vi "MC_7_12c_JW.vi"() -> ()   [LabVIEW 2011]
uses:
  <vilib>/Utility/file.llb/Read From Spreadsheet File (string).vi
  <vilib>/regexp/Match Regular Expression.xnode
  <vilib>/Utility/file.llb/Write To Spreadsheet File (string).vi
  <vilib>/Utility/file.llb/Write To Spreadsheet File (DBL).vi
  <vilib>/Utility/inputDevices.llb/keyboardAcquire.vi
panel:
  out "Rec: Temp":dbl
  out "Date Created":string
  out "Comments":string
  out "Folder Index":dbl caption="Length"
  out "Current \nRecord":string[](array[string])
  out "Transformer \nHeaders":string[](array[string])
  out "Current Device ID":string
  out "Column":string
  out "Row":string
  out "Rec: Concentration":dbl
  out "Rec: Solvent":string
  out "Rec: Method":string
  in  "?":T1(tab)
  out "Rec: Material":string
  in  "Treatment Concentration (mM):":dbl=30.0
  in  "Surface Treatment:":string
  in  "# Drops*:":dbl=inf
  in  "Solution Temp (C):":dbl=55.0
  in  "Relative Humidity (%):":dbl=nan
  in  "Room Temp (F):":dbl=nan
  in  "Time (s):":dbl=80.0
  out "Accel (RPM/s):":dbl
  in  "RPM:":dbl=1000.0
  in  "Wait Time (s):":dbl=10.0
  in  "Sample #:":dbl=1.0
  in  "Fabricator:":string="Jeremy"
  in  "Data File":path
  out "Data Folder":path
  in  "Image Folder":path
  out "Image File":path=path "D:/UserData/Desktop/Jeremy/WFU/Research/Programs/VI mods/Image Not Found.png"
  in  "Ramp (s):":dbl=3.0
  out "Calc: Trap Density-STS":dbl format="%#_4e"
  out "New: Trap Density-STS":dbl format="%#_4e"
  out "Rec: Trap Density-STS":dbl caption="Trap Density-STS" format="%#_4e"
  out "Calc: Trap Density-VT":dbl format="%#_4e"
  out "New: Trap Density-VT":dbl format="%#_4e"
  out "Rec: Trap Density-VT":dbl caption="Trap Density-VT" format="%#_4e"
  out "Calc: Onset V":dbl
  out "New: Onset":dbl
  out "Rec: Onset V":dbl caption="Onset V"
  out "Calc: Mobility-Lin":dbl format="%#_4e"
  out "New: Mobility-Lin":dbl format="%#_4e"
  out "Rec: Mobility-Lin":dbl caption="Mobility-Lin" format="%#_4e"
  out "Calc: Mobility-Sat":dbl format="%#_4e"
  out "Rec: Length":dbl caption="Length"
  out "Rec: Width":dbl caption="Width"
  out "Rec: Dielectric (d)":dbl caption="Dielectric (d)"
  out "XY Graph":cluster{dbl[], dbl[]}[](graph)
  in  "NumPts":dbl=5.0
  in  "Cancel Button":bool
  in  "Next Button":bool
  in  "Previous Button":bool
  in  "Up Button":bool
  in  "Down Button":bool
  out "Data Name":string
  in  "Save Changes?":bool
  in  "New: Dielectric":dbl
  in  "New: Length":dbl
  in  "New: Width":dbl
  out "New: Mobility-Sat":dbl format="%#_4e"
  in  "Slide":dbl(slide) step=1.0 scale=-14.3..84.0 scale format="%#_1p"
  in  "Blank Button":bool
  in  "Zoom":i16(slide)=-3 scale=-5.0..5.0
  out "Image Out 2":T2(plugin-control)
  out "Image Out":T2(plugin-control)
  in  "Magnification":u16(ring) items=["5x", "10x", "20x", "50x", "80x"]
  out "Total Width":dbl
  out "Distances":dbl[](array[numeric])
  in  "Undo Button":bool
  in  "Remove Button":bool
  out "Rec: Mobility-Sat":dbl caption="Mobility-Sat" format="%#_4e"
  out "Index":string
  out "Image Name":string
  in  "Export":bool
  out "Calc: VT":dbl
  out "New: VT":dbl
  in  "Manual":bool
  out "XY Graph 2":cluster{dbl[], dbl[]}[](graph)
  in  "Next Button 2":bool
  in  "Previous Button 2":bool
  in  "Slide 2":dbl(slide) step=1.0 scale=-1.0..82.0 scale format="%#_1p"
  out "Calc: STS":dbl
  out "New: STS":dbl
  in  "NumPts 2":dbl=5.0 caption="NumPts"
  out "Rec: VT":dbl caption="Threshold V"
  out "Rec: STS":dbl caption="STS"
  out "Rec: On/Off":dbl caption="On/Off" format="%#_3e"
  in  "Save Changes? 2":bool
  in  "Save Changes? 3":bool
  out "Date Recorded":string="Date Recorded"
  out "String":string
  in  "No Image":path=path "D:/UserData/Desktop/Jeremy/WFU/Research/Programs/VI mods/Image Not Found.png"
  in  "Project":path=path "D:/UserData/Desktop/Jeremy/WFU/Research/Programs/Mega Awesome/DeviceData.opj"
  out "Index 2":dbl
  out "Array 8":dbl[](array[numeric])
  out "Array 7":dbl[](array[numeric])
  out "ROI Descriptor out":T3 {"Contours"."Type" items=["No Selection", "Point", "Line", "Rectangle", "Oval", "Polygon", "Freehand Region", "Annulus", "Unused2", "Unused3", "Broken Line", "Freehand Line", "Rotated Rectangle"]}
  out "ROI Descriptor":T3 {"Contours"."Type" items=["No Selection", "Point", "Line", "Rectangle", "Oval", "Polygon", "Freehand Region", "Annulus", "Unused2", "Unused3", "Broken Line", "Freehand Line", "Rotated Rectangle"]}
  out "Numeric 3":dbl
  out "Array 6":dbl[][](array[numeric])
  out "Cluster":T4
  out "Array 5":dbl[](array[numeric])
  out "Array 4":dbl[](array[numeric])
  out "Array 3":dbl[](array[numeric])
  out "Numeric 2":dbl
  out "Numeric":dbl
  out "Array 2":dbl[](array[numeric])
  out "Array":dbl[](array[numeric])
  out "Device Index":dbl
  out "Table Control 2":string[][](table)
  out "Table Control":string[][](table)
  in  "Row Start":dbl=20.0
  # "Data Locations"
  # "Data Location"
  # "Image Location"
  # "Sample Properties"
  # "*     Inf = Full coverage\n   NaN = Unknown or Not Applicable"
  # "Recorded"
  # "Calculated"
  # "Re-Calculated"
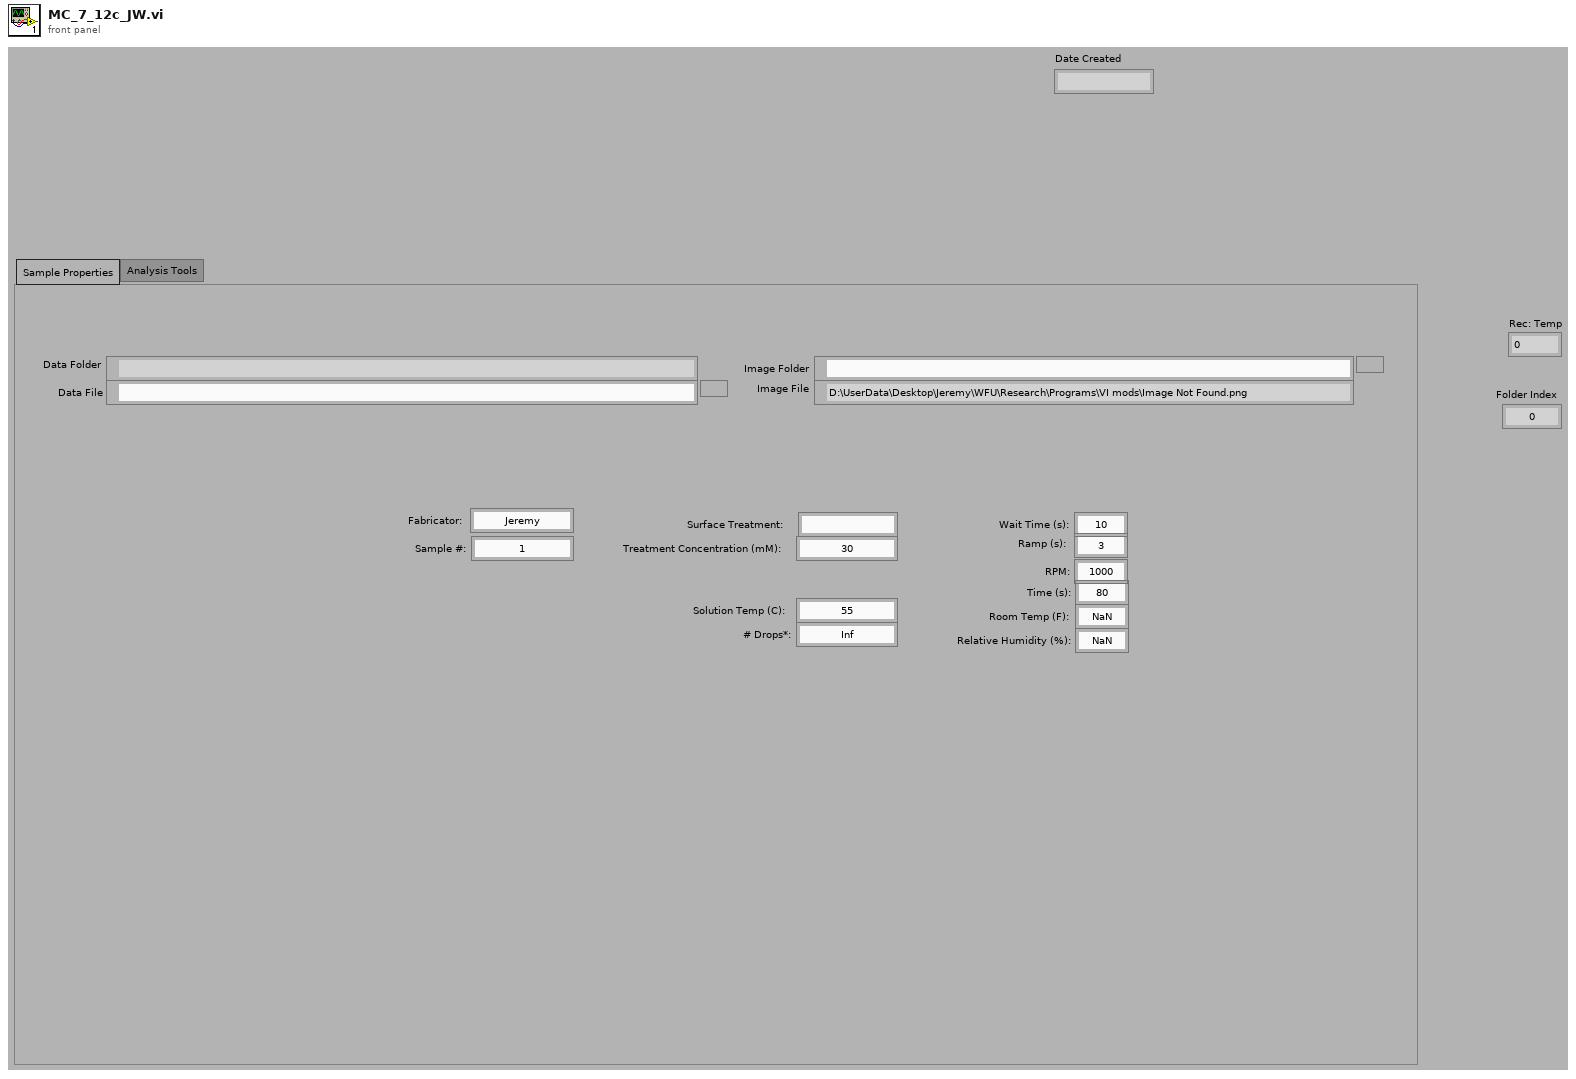
[diagram p1: front panel]
types:
  T1 = enum32{"Sample Properties", "Analysis Tools", "Current Database"}
  T2 = typedef "IMAQ Image.ctl" = refnum<image>
  T3 = typedef "ROI Descriptor" = cluster{"Global Rectangle":i32[], "Contours":cluster{"ID":enum32{"External", "Internal"}, "Type":u32, "Coordinates":i32[]}[]}
  T4 = cluster{"Numeric":dbl, "Numeric 2":dbl, "Numeric 3":dbl, "Numeric 4":dbl}
  T5 = cluster{"Mobility-Sat":dbl, "Moblitity-Lin":dbl, "On/Off":dbl, "Threshold Voltage":dbl, "Onset Voltage":dbl, "STS":dbl, "Trap Density-VT":dbl, "Trap Density-STS":dbl}
  T6 = cluster{"Date Recorded":string, "Index":string, "Length":dbl, "Width":dbl, "Sample Temp":dbl}
  T7 = cluster{"Date Created":string, "Material":string, "Solvent":string, "Concentration":dbl, "Method":string, "Dielectric (nm)":dbl, "Treatment":string, "Comments":string}
  T8 = cluster{"[0]":cluster{dbl[], dbl[]}, "[1]":cluster{dbl[], dbl[]}, "[2]":cluster{dbl[], dbl[]}, "[3]":cluster{dbl[], dbl[]}, "[4]":cluster{dbl[], dbl[]}, "[5]":cluster{dbl[], dbl[]}, "[6]":cluster{dbl[], dbl[]}, "[7]":cluster{dbl[], dbl[]}, "[8]":cluster{dbl[], dbl[]}}
  T9 = cluster{"Global Rectangle":i32[], "Contours":cluster{"Contour Type":u32, "ROI Type":u32, "Points":i32[]}[]}
  T10 = typedef "LVBoundsTypeDef.ctl" = cluster{"Width":u32, "Height":u32}
  T11 = enum16{"0", "1", "2", "3", "4", "5", "6", "7", "8", "9", "A", "B", "C", "D", "E", "F", "G", "H", "I", "J", "K", "L", "M", "N", "O", "P", "Q", "R", "S", "T", "U", "V", "W", "X", "Y", "Z", "F1", "F2", "F3", "F4", "F5", "F6", "F7", "F8", "F9", "F10", "F11", "F12", "F13", "F14", "F15", "ADD", "BACK", "BACKSLASH", "CAPITAL", "COMMA", "DECIMAL", "DELETE", "DIVIDE", "DOWN", "END", "EQUALS", "ESCAPE", "GRAVE (`)", "HOME", "INSERT", "LBRACKET", "LCONTROL", "LEFT", "L ALT", "LSHIFT", "LWIN", "MINUS", "MULTIPLY", "NEXT", "NUMLOCK", "NUMPAD_0", "NUMPAD_1", "NUMPAD_2", "NUMPAD_3", "NUMPAD_4", "NUMPAD_5", "NUMPAD_6", "NUMPAD_7", "NUMPAD_8", "NUMPAD_9", "PAUSE", "PERIOD", "PRIOR (PG UP)", "RBRACKET", "RCONTROL", "RETURN", "RIGHT", "R ALT", "RSHIFT", "RWIN", "SCROLL", "SEMICOLON", "SLASH", "SPACE", "SUBTRACT", "TAB", "UP", "ENTER (num pad)", "' (quote)"}[]
  T12 = cluster{"Contour Type":u32, "ROI Type":u32, "Points":i32[]}[]
  T13 = cluster{i32[], cluster{"Contour Type":u32, "ROI Type":u32, "Points":i32[]}[]}
  T14 = enum16{"0", "1", "2", "3", "4", "5", "6", "7", "8", "9", "A", "B", "C", "D", "E", "F", "G", "H", "I", "J", "K", "L", "M", "N", "O", "P", "Q", "R", "S", "T", "U", "V", "W", "X", "Y", "Z", "F1", "F2", "F3", "F4", "F5", "F6", "F7", "F8", "F9", "F10", "F11", "F12", "F13", "F14", "F15", "ADD", "BACK", "BACKSLASH", "CAPITAL", "COMMA", "DECIMAL", "DELETE", "DIVIDE", "DOWN", "END", "EQUALS", "ESCAPE", "GRAVE (`)", "HOME", "INSERT", "LBRACKET", "LCONTROL", "LEFT", "L ALT", "LSHIFT", "LWIN", "MINUS", "MULTIPLY", "NEXT", "NUMLOCK", "NUMPAD_0", "NUMPAD_1", "NUMPAD_2", "NUMPAD_3", "NUMPAD_4", "NUMPAD_5", "NUMPAD_6", "NUMPAD_7", "NUMPAD_8", "NUMPAD_9", "PAUSE", "PERIOD", "PRIOR (PG UP)", "RBRACKET", "RCONTROL", "RETURN", "RIGHT", "R ALT", "RSHIFT", "RWIN", "SCROLL", "SEMICOLON", "SLASH", "SPACE", "SUBTRACT", "TAB", "UP", "ENTER (num pad)", "' (quote)"}
  T15 = cluster{string, sgl, bool, bool, bool, bool, bool, bool, i32}
  T16 = cluster{i32, cluster{string, sgl, bool, bool, bool, bool, bool, bool, i32}, i32, i32}
  T17 = cluster{"Contour Type":u32, "ROI Type":u32, "Points":i32[]}
  T18 = cluster{"Points[0]":i32, "Points[1]":i32, "Points[2]":i32, "Points[3]":i32, "Points[4]":i32, "Points[5]":i32, "Points[6]":i32, "Points[7]":i32, "Points[8]":i32}
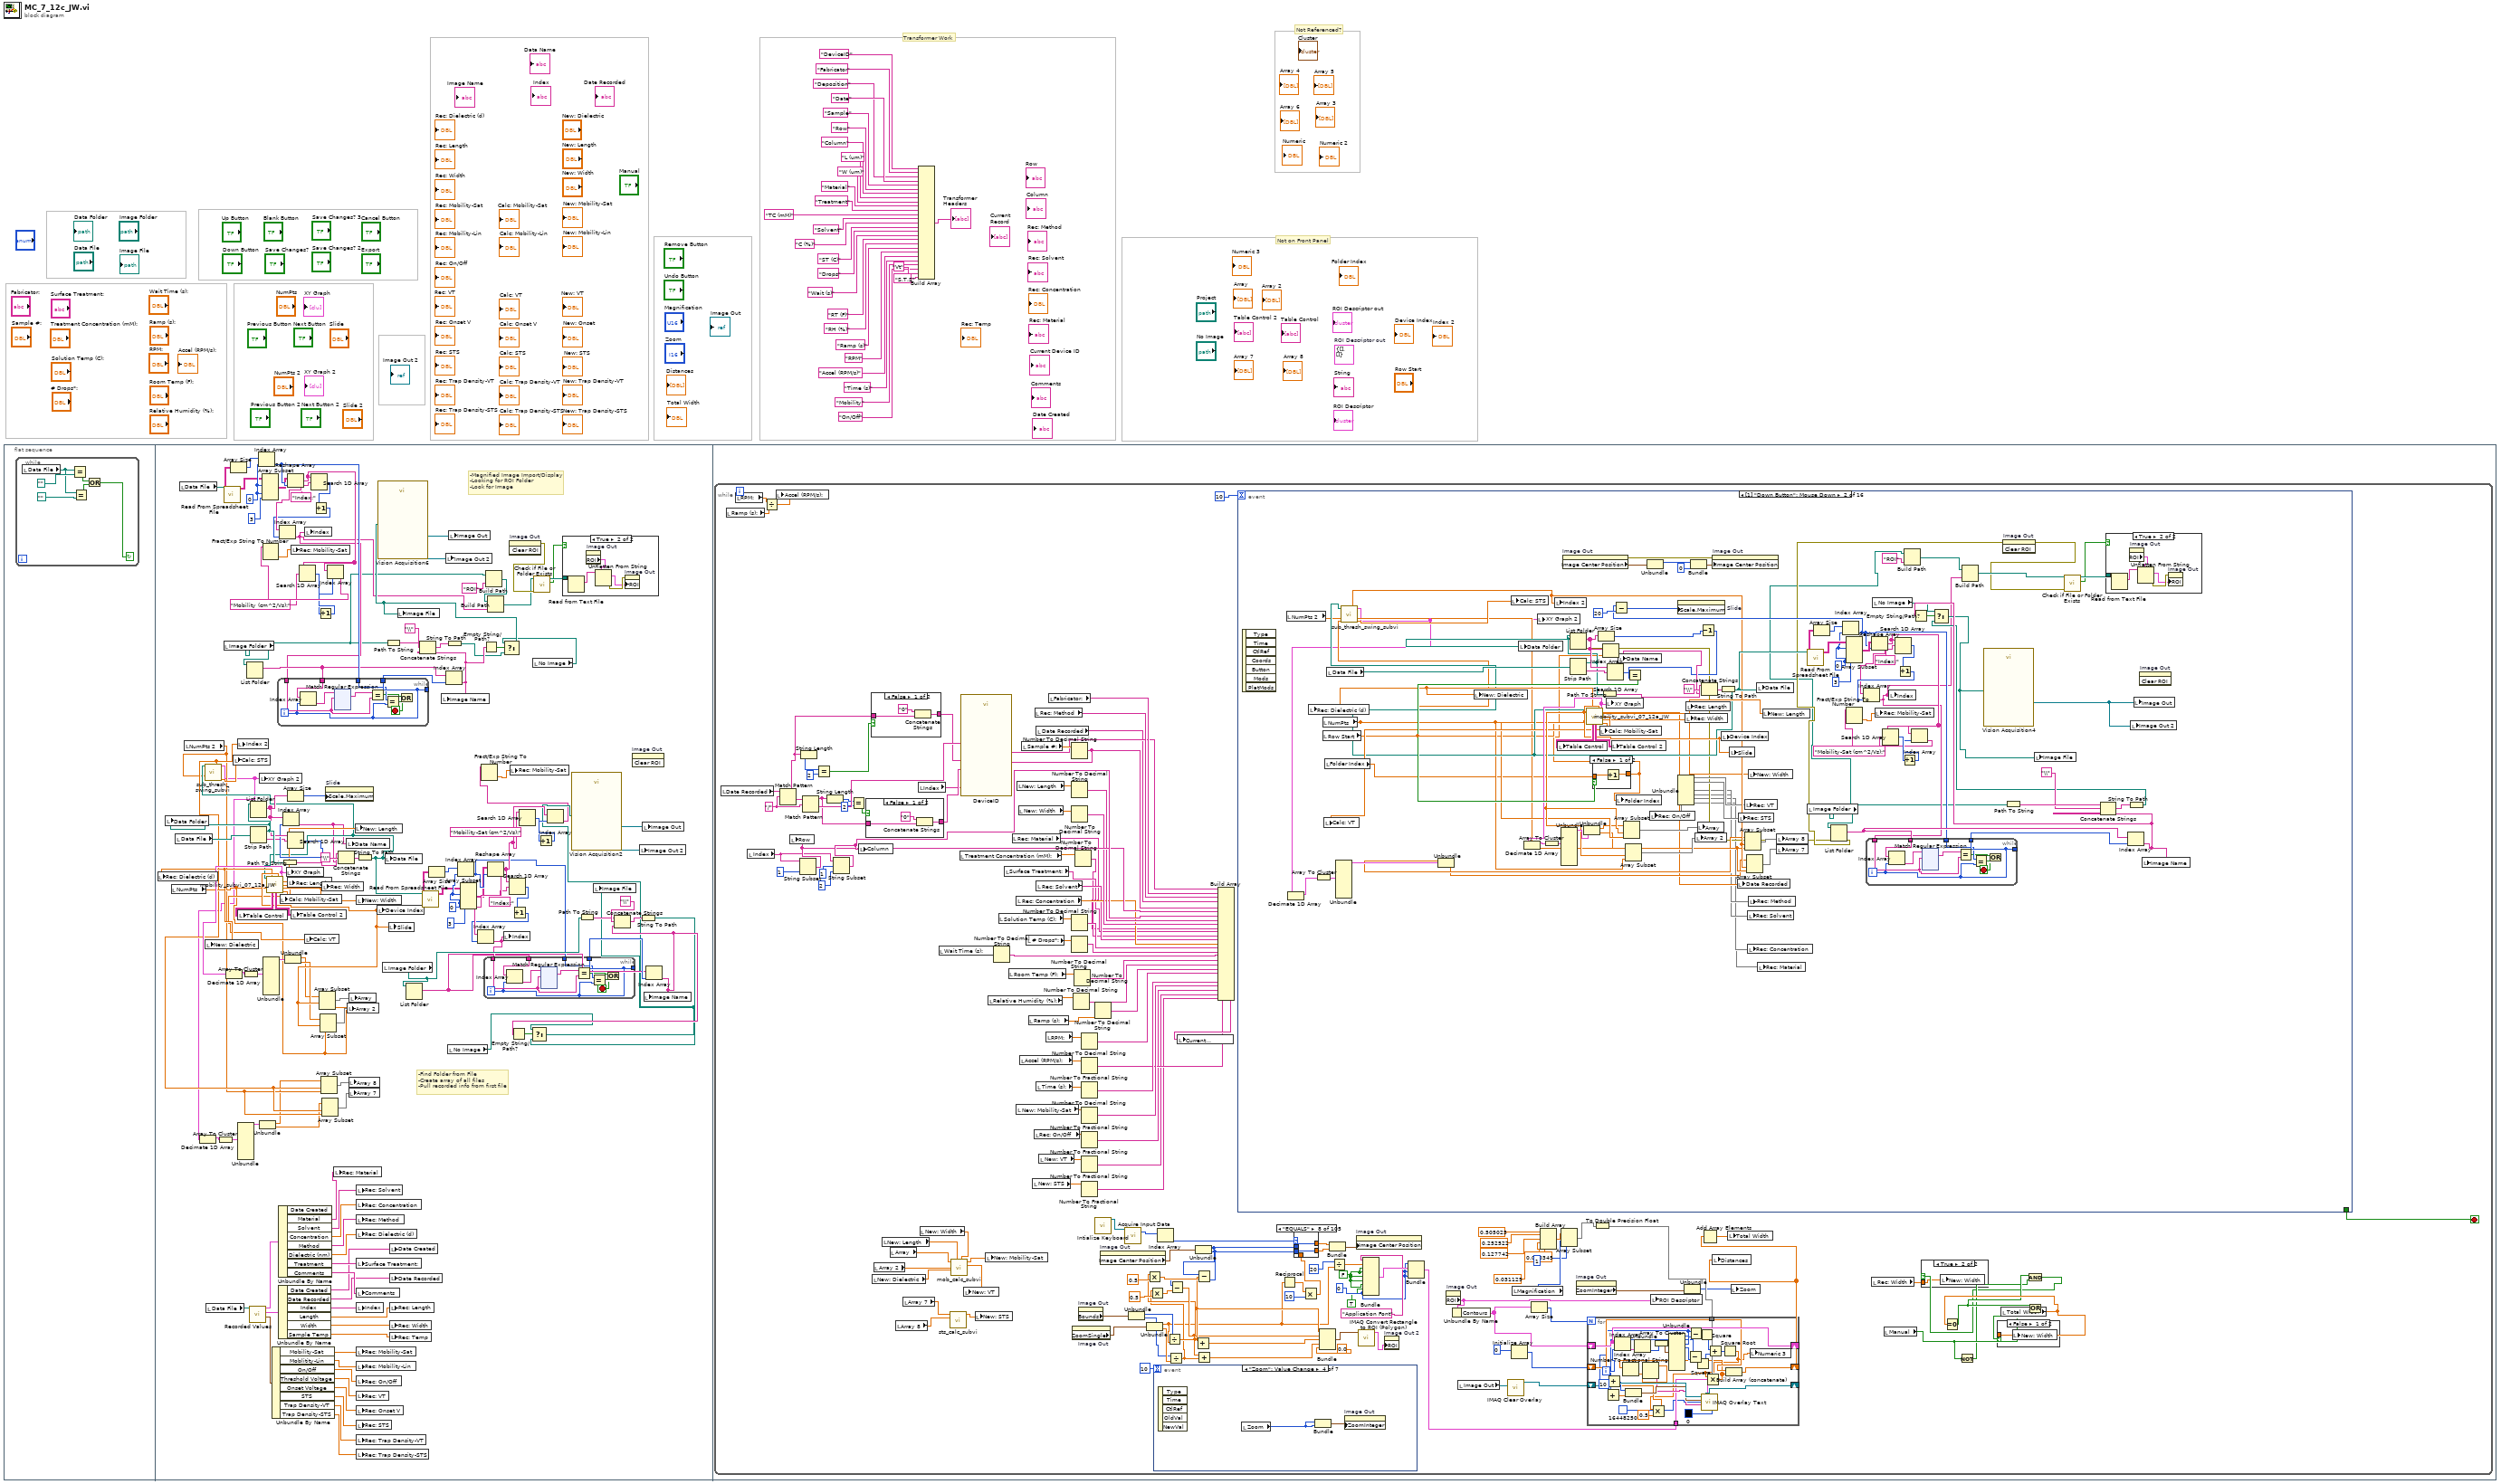
[diagram p0: block diagram]
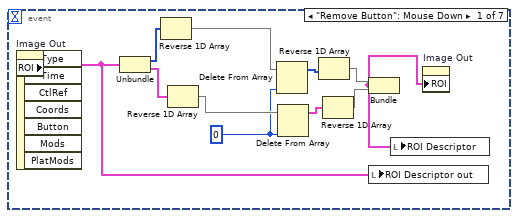
[diagram p7: hidden frame]
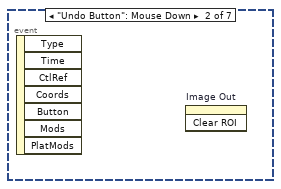
[diagram p8: hidden frame]
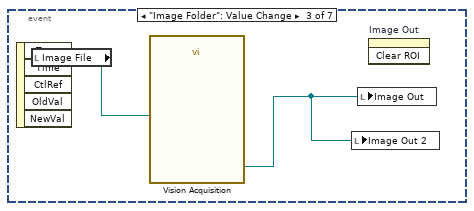
[diagram p9: hidden frame]
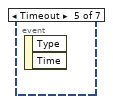
[diagram p10: hidden frame]
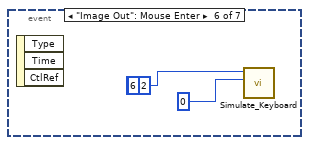
[diagram p11: hidden frame]
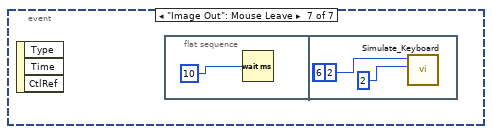
[diagram p12: hidden frame]
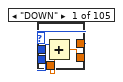
[diagram p13: hidden frame]
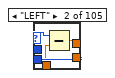
[diagram p14: hidden frame]
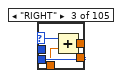
[diagram p15: hidden frame]
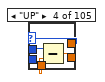
[diagram p16: hidden frame]
diagram:
  (unwired) T3 {"Global Rectangle"=[], "Contours"=[]}  # ROI Descriptor out
  # "Not Referenced?"
  # "Transformer Work"
  # "Not on Front Panel"
  n1 = flat-sequence {
    frame #0 {
      n2 = while {
        stop <- w29 continue-if-true
        n3 = local read "Data File"() -> (w31:path)
        n4 = Equal?(x=w31, y=path "") -> (x = y?=w33:bool)
        n5 = Equal?(x=w31, y=path "") -> (x = y?=w32:bool)
        n6 = Or(x=w33, y=w32) -> (x .or. y?=w29:bool)
      }
    }
    frame #1 {
      w116 = 0
      w145 = 0
      # "-Find Folder from File\n-Create array of all files\n-Pull recorded info from first file"
      # "-Magnified Image Import/Display\n-Looking for ROI Folder\n-Look for Image"
      n7 = local read "NumPts"() -> (w92:dbl)
      n8 = local read "Data File"() -> (w120:path)
      n9 = local read "Data File"() -> (w140:path)
      n10 = local read "NumPts 2"() -> (w87:dbl)
      n11 = local read "Data File"() -> (w59:path)
      n12 = call-poly <vilib>:"Read From Spreadsheet File.vi"("file path (dialog if empty)"=w140) -> ("all rows"=w143:string[][])  [unwired: 6 in, 4 out]
      n13 = local read "Image Folder"() -> (w62:path)
      n14 = Array Size(array=w143) -> (size(s)=w144:i32[])
      n15 = List Folder(path=w62) -> (filenames=w149:string[])  [unwired: 3 in, 3 out]
      n16 = call "Recorded Values.vi"("Path"=w59) -> ("Recorded Char"=w57:T5, "Recorded Prop"=w56:T6, "Fabrication Prop"=w58:T7)  [unwired: 8 in]
      n17 = Strip Path(path=w120) -> (stripped path=w121:path, name=w103:string)
      n18 = local write "Data Folder"(w121) -> ()
      n19 = List Folder(path=w121) -> (filenames=w110:string[])  [unwired: 3 in, 3 out]
      n20 = Index Array(array=w144, index=w145) -> (element=w151:i32)
      n21 = Array Subset(array=w143, index (row)=w145, index (col)=w145, length (col)=3) -> (w142:string[][])  [unwired: 1 in]
      n22 = Unbundle By Name(w57) -> ("Mobility-Sat"=w42:dbl, "Moblitity-Lin"=w41:dbl, "On/Off"=w40:dbl, "Threshold Voltage"=w39:dbl, "Onset Voltage"=w38:dbl, "STS"=w37:dbl, "Trap Density-VT"=w36:dbl, "Trap Density-STS"=w35:dbl)
      n23 = Unbundle By Name(w58) -> ("Material"=w55:string, "Solvent"=w54:string, "Concentration"=w53:dbl, "Method"=w52:string, "Dielectric (nm)"=w51:dbl, "Treatment"=w50:string, "Comments"=w49:string)  [unwired: 1 out]
      n24 = Unbundle By Name(w56) -> ("Date Created"=w48:string, "Date Recorded"=w47:string, "Index"=w46:string, "Length"=w45:dbl, "Width"=w44:dbl, "Sample Temp"=w43:dbl)
      n25 = Path To String(path=w121) -> (string=w102:string)
      n26 = Reshape Array(w142, w151) -> (w161:string[])
      n27 = Array Size(array=w110) -> (size(s)=w111:i32)
      n28 = Search 1D Array(1D array=w110, element=w103) -> (index of element=w109:i32)  [unwired: 1 in]
      n29 = Index Array(array=w110, index=w109) -> (element=w61:string)
      n30 = Search 1D Array(1D array=w161, element="Mobility (cm^2/Vs):") -> (index of element=w156:i32)  [unwired: 1 in]
      n31 = Search 1D Array(1D array=w161, element="Index:") -> (index of element=w148:i32)  [unwired: 1 in]
      n32 = Increment(x=w148) -> (x+1=w147:i32)
      n33 = Index Array(array=w161, index=w147) -> (element=w63:string)
      n34 = while {
        tunnel: w149 -> [w294]
        tunnel: w63 -> [w292]
        tunnel: [w291] -> _
        tunnel: [w291] -> w150
        tunnel: w151 -> [w290]
        i -> [w291]
        stop <- w287 stop-if-true
        n35 = Index Array(array=w294, index=w291) -> (element=w295:string)
        n36 = xnode "Match Regular Expression"("input string"=w295, "regular expression"=w292) -> ("whole match"=w293:string)  [unwired: 4 in, 4 out]
        n37 = Equal?(x=w293, y=w292) -> (x = y?=w289:bool)
        n38 = Equal?(x=w290, y=w291) -> (x = y?=w288:bool)
        n39 = Or(x=w289, y=w288) -> (x .or. y?=w287:bool)
      }
      n40 = local write "Index"(w63) -> ()
      n41 = Increment(x=w156) -> (x+1=w157:i32)
      n42 = property on="Slide" class="Slide (strict)"("Scale.Maximum"=w111) -> ()  [unwired: 2 in, 2 out]
      n43 = Index Array(array=w161, index=w157) -> (element=w159:string)
      n44 = Fract/Exp String To Number(string=w159) -> (number=w160:dbl)  [unwired: 3 in, 1 out]
      n45 = local write "Rec: Mobility-Sat"(w160) -> ()
      n46 = local write "Rec: Material"(w55) -> ()
      n47 = Concatenate Strings(w102, "\\", w61) -> (w104:string)
      n48 = local write "Data Name"(w61) -> ()
      n49 = local write "Rec: Solvent"(w54) -> ()
      n50 = local write "Rec: Concentration"(w53) -> ()
      n51 = local write "Rec: Method"(w52) -> ()
      n52 = local write "Rec: Dielectric (d)"(w51) -> ()
      n53 = local write "Surface Treatment:"(w50) -> ()
      n54 = local write "Comments"(w49) -> ()
      n55 = local write "Index"(w46) -> ()
      n56 = local write "Rec: Mobility-Sat"(w42) -> ()
      n57 = local write "Rec: Mobility-Lin"(w41) -> ()
      n58 = local write "Rec: On/Off"(w40) -> ()
      n59 = local write "Rec: VT"(w39) -> ()
      n60 = local write "Rec: Onset V"(w38) -> ()
      n61 = local write "Rec: STS"(w37) -> ()
      n62 = local write "Rec: Trap Density-VT"(w36) -> ()
      n63 = local write "Rec: Trap Density-STS"(w35) -> ()
      n64 = String To Path(string=w104) -> (path=w93:path)
      n65 = call "sub_thresh_swing_subvi.vi"("Path"=w93, "NumPts"=w87) -> ("Index"=w88:dbl, "XY Graph"=w83:cluster{dbl[], dbl[]}[], "Sub Threshold Swing"=w94:dbl)  [unwired: 9 in, 2 out]
      n66 = Decimate 1D Array(w83) -> (w84:cluster{dbl[], dbl[]}[])  [unwired: 1 out]
      n67 = Array To Cluster(array=w84) -> (cluster=w86:T8)
      n68 = local write "Calc: STS"(w94) -> ()
      n69 = local write "Index 2"(w88) -> ()
      n70 = Unbundle(w86) -> ("[0]"=w85:cluster{dbl[], dbl[]})  [unwired: 8 out]
      n71 = local write "XY Graph 2"(w83) -> ()
      n72 = Unbundle(w85) -> (w81:dbl[], w80:dbl[])
      n73 = call "mobility_subvi_07_12a_JW.vi"("Path"=w93, "NumPts"=w92) -> ("Dielectric (d)"=w98:dbl, "Index"=w99:dbl, "XY Graph"=w139:cluster{dbl[], dbl[]}[], "Length"=w97:dbl, "Vt"=w95:dbl, "Width"=w96:dbl, "Table Control"=w106:string[][], "Table Control 2"=w107:string[][], "Mobility"=w108:dbl)  [unwired: 4 in, 1 out]
      n74 = local write "Rec: Dielectric (d)"(w98) -> ()
      n75 = local write "New: Dielectric"(w98) -> ()
      n76 = Decimate 1D Array(w139) -> (w138:cluster{dbl[], dbl[]}[])  [unwired: 1 out]
      n77 = local write "Table Control"(w106) -> ()
      n78 = Array To Cluster(array=w138) -> (cluster=w136:T8)
      n79 = Unbundle(w136) -> ("[0]"=w137:cluster{dbl[], dbl[]})  [unwired: 8 out]
      n80 = local write "Calc: Mobility-Sat"(w108) -> ()
      n81 = Unbundle(w137) -> (w82:dbl[], w89:dbl[])
      n82 = local write "XY Graph"(w139) -> ()
      n83 = local write "Rec: Length"(w97) -> ()
      n84 = local write "Table Control 2"(w107) -> ()
      n85 = local write "Calc: VT"(w95) -> ()
      n86 = Array Subset(array=w82, index=w99, length=w92) -> (w100:dbl[])
      n87 = Array Subset(array=w89, index=w99, length=w92) -> (w101:dbl[])
      n88 = Array Subset(array=w81, index=w88, length=w87) -> (w91:dbl[])
      n89 = local write "Rec: Width"(w96) -> ()
      n90 = Array Subset(array=w80, index=w88, length=w87) -> (w90:dbl[])
      n91 = local write "Array 2"(w101) -> ()
      n92 = local write "Array 8"(w91) -> ()
      n93 = local write "Array 7"(w90) -> ()
      n94 = local write "Array"(w100) -> ()
      n95 = local write "New: Length"(w97) -> ()
      n96 = local write "New: Width"(w96) -> ()
      n97 = local write "Device Index"(w99) -> ()
      n98 = local read "Image Folder"() -> (w127:path)
      n99 = local write "Data File"(w93) -> ()
      n100 = Path To String(path=w62) -> (string=w153:string)
      n101 = local write "Slide"(w99) -> ()
      n102 = local write "Date Created"(w48) -> ()
      n103 = local write "Date Recorded"(w47) -> ()
      n104 = local write "Rec: Length"(w45) -> ()
      n105 = local write "Rec: Width"(w44) -> ()
      n106 = local write "Rec: Temp"(w43) -> ()
      n107 = List Folder(path=w127) -> (filenames=w123:string[])  [unwired: 3 in, 3 out]
      n108 = call-poly <vilib>:"Read From Spreadsheet File.vi"("file path (dialog if empty)"=w93) -> ("all rows"=w114:string[][])  [unwired: 6 in, 4 out]
      n109 = Array Size(array=w114) -> (size(s)=w115:i32[])
      n110 = Index Array(array=w149, index=w150) -> (element=w79:string)
      n111 = Concatenate Strings(w153, "\\", w79) -> (w154:string)
      n112 = local write "Image Name"(w79) -> ()
      n113 = String To Path(string=w154) -> (path=w77:path)
      n114 = local read "No Image"() -> (w71:path)
      n115 = Index Array(array=w115, index=w116) -> (element=w126:i32)
      n116 = Array Subset(array=w114, index (row)=w116, index (col)=w116, length (col)=3) -> (w113:string[][])  [unwired: 1 in]
      n117 = Empty String/Path?(string/path=w79) -> (empty?=w78:bool)
      n118 = Build Path(base path=w62, name or relative path="ROI") -> (appended path=w65:path)
      n119 = Build Path(base path=w65, name or relative path=w63) -> (appended path=w64:path)
      n120 = Reshape Array(w113, w126) -> (w135:string[])
      n121 = invoke on="Image Out" class="ImageControl" method="Clear ROI"() -> (error out=w69:errorcluster)  [unwired: 3 in, 2 out]
      n122 = Search 1D Array(1D array=w135, element="Index:") -> (index of element=w119:i32)  [unwired: 1 in]
      n123 = Increment(x=w119) -> (x+1=w118:i32)
      n124 = Index Array(array=w135, index=w118) -> (element=w124:string)
      n125 = while {
        tunnel: w123 -> [w174]
        tunnel: w124 -> [w172]
        tunnel: [w171] -> _
        tunnel: [w171] -> w125
        tunnel: w126 -> [w170]
        i -> [w171]
        stop <- w167 stop-if-true
        n126 = Index Array(array=w174, index=w171) -> (element=w175:string)
        n127 = xnode "Match Regular Expression"("input string"=w175, "regular expression"=w172) -> ("whole match"=w173:string)  [unwired: 4 in, 4 out]
        n128 = Equal?(x=w173, y=w172) -> (x = y?=w169:bool)
        n129 = Equal?(x=w170, y=w171) -> (x = y?=w168:bool)
        n130 = Or(x=w169, y=w168) -> (x .or. y?=w167:bool)
      }
      n131 = local write "Index"(w124) -> ()
      n132 = Search 1D Array(1D array=w135, element="Mobility-Sat (cm^2/Vs):") -> (index of element=w131:i32)  [unwired: 1 in]
      n133 = local read "No Image"() -> (w70:path)
      n134 = Select(t=w70, s=w78, f=w77) -> (s? t:f=w76:path)
      n135 = call "Vision Acquisition6"("Image Path"=w76) -> ("Image Out"=w152:T2)  [unwired: 25 in, 1 out]
      n136 = local write "Image File"(w76) -> ()
      n137 = local write "Image Out 2"(w152) -> ()
      n138 = local write "Image Out"(w152) -> ()
      n139 = call <vilib>:"Check if File or Folder Exists.vi"("error in (no error)"=w69, "path"=w64) -> ("file or folder exists?"=w67:bool, "dup path"=w68:path)  [unwired: 7 in, 1 out]
      n140 = Increment(x=w131) -> (x+1=w132:i32)
      n141 = Index Array(array=w135, index=w132) -> (element=w60:string)
      n142 = Fract/Exp String To Number(string=w60) -> (number=w134:dbl)  [unwired: 3 in, 1 out]
      n143 = local write "Rec: Mobility-Sat"(w134) -> ()
      n144 = case shown="True" w67 {
        tunnel: w68 -> [_ w162]
        frame False {
        }
        frame True {
          n145 = Read from Text File(file (use dialog)=w162) -> (text=w166:string)  [unwired: 3 in, 3 out]
          n146 = property on="Image Out" class="ImageControl"() -> ("ROI"=w163:T9)  [unwired: 2 in, 2 out]
          n147 = Unflatten From String(type=w163, binary string=w166) -> (value=w164:T9, error out=w165:errorcluster)  [unwired: 3 in, 1 out]
          n148 = property on="Image Out" class="ImageControl"(error in=w165, "ROI"=w164) -> ()  [unwired: 1 in, 2 out]
        }
      }
      n149 = Path To String(path=w127) -> (string=w128:string)
      n150 = invoke on="Image Out" class="ImageControl" method="Clear ROI"() -> ()  [unwired: 3 in, 3 out]
      n151 = Index Array(array=w123, index=w125) -> (element=w74:string)
      n152 = Empty String/Path?(string/path=w74) -> (empty?=w75:bool)
      n153 = Concatenate Strings(w128, "\\", w74) -> (w129:string)
      n154 = String To Path(string=w129) -> (path=w73:path)
      n155 = Select(t=w71, s=w75, f=w73) -> (s? t:f=w72:path)
      n156 = call "Vision Acquisition2"("Image Path"=w72) -> ("Image Out"=w122:T2)  [unwired: 25 in, 1 out]
      n157 = local write "Image File"(w72) -> ()
      n158 = local write "Image Out 2"(w122) -> ()
      n159 = local write "Image Out"(w122) -> ()
      n160 = local write "Image Name"(w74) -> ()
    }
    frame #2 {
      n161 = while {
        stop <- w553 stop-if-true
        w439 = "/"
        w503 = FALSE
        w501 = 0
        n162 = local read "Date Recorded"() -> (w442:string)
        n163 = local read "Ramp (s):"() -> (w408:dbl)
        n164 = local read "RPM:"() -> (w409:dbl)
        n165 = local read "Index"() -> (w411:string)
        n166 = Divide(x=w409, y=w408) -> (x/y=w407:dbl)
        n167 = local write "Accel (RPM/s):"(w407) -> ()
        n168 = Match Pattern(string=w442, regular expression=w439) -> (before substring=w433:string, after substring=w440:string)  [unwired: 1 in, 2 out]
        n169 = String Subset(string=w411, length (rest)=1) -> (substring=w467:string)  [unwired: 1 in]
        n170 = local write "Row"(w467) -> ()
        n171 = String Length(string=w433) -> (length=w436:i32)
        n172 = Match Pattern(string=w440, regular expression=w439) -> (before substring=w427:string, after substring=w438:string)  [unwired: 1 in, 2 out]
        n173 = Equal?(x=w436, y=2) -> (x = y?=w434:bool)
        n174 = String Length(string=w427) -> (length=w429:i32)
        n175 = String Subset(string=w411, offset (0)=1, length (rest)=2) -> (substring=w468:string)
        n176 = Equal?(x=w429, y=2) -> (x = y?=w431:bool)
        n177 = local write "Column"(w468) -> ()
        n178 = case shown="False" w431 {
          tunnel: w427 -> [w555 w557]
          tunnel: [w554 w557] -> w428
          frame False {
            n179 = Concatenate Strings("0", w555) -> (w554:string)
          }
          frame True {
          }
        }
        n180 = case shown="False" w434 {
          tunnel: w433 -> [w559 w561]
          tunnel: [w558 w561] -> w432
          frame False {
            n181 = Concatenate Strings("0", w559) -> (w558:string)
          }
          frame True {
          }
        }
        n182 = local read "New: Dielectric"() -> (w491:dbl)
        n183 = local read "Array 2"() -> (w487:dbl[])
        n184 = local read "New: Length"() -> (w489:dbl)
        n185 = local read "Array"() -> (w488:dbl[])
        n186 = local read "Array 8"() -> (w483:dbl[])
        n187 = local read "Array 7"() -> (w484:dbl[])
        n188 = local read "Index"() -> (w426:string)
        n189 = local read "New: Width"() -> (w492:dbl)
        n190 = local read "Wait Time (s):"() -> (w472:dbl)
        n191 = call "sts_calc_subvi.vi"("Array 2"=w483, "Array"=w484) -> ("STS"=w485:dbl)  [unwired: 9 in]
        n192 = call "mob_calc_subvi.vi"("Width"=w492, "Length"=w489, "Dielectric (d)"=w491, "Array 2"=w487, "Array"=w488) -> ("Vt"=w486:dbl, "Mobility"=w490:dbl)  [unwired: 4 in, 1 out]
        n193 = local read "Treatment Concentration (mM):"() -> (w419:dbl)
        n194 = local write "New: VT"(w486) -> ()
        n195 = local write "New: STS"(w485) -> ()
        n196 = local write "New: Mobility-Sat"(w490) -> ()
        n197 = local read "Relative Humidity (%):"() -> (w416:dbl)
        n198 = Number To Decimal String(number=w472) -> (decimal integer string=w473:string)  [unwired: 1 in]
        n199 = local read "Solution Temp (C):"() -> (w461:dbl)
        n200 = local read "Surface Treatment:"() -> (w418:string)
        n201 = local read "Room Temp (F):"() -> (w465:dbl)
        n202 = local read "Rec: Material"() -> (w414:string)
        n203 = local read "Rec: Concentration"() -> (w421:dbl)
        n204 = local read "New: Mobility-Sat"() -> (w454:dbl)
        n205 = local read "New: Length"() -> (w425:dbl)
        n206 = local read "New: Width"() -> (w424:dbl)
        n207 = local read "Accel (RPM/s):"() -> (w452:dbl)
        n208 = local read "Sample #:"() -> (w444:dbl)
        n209 = local read "# Drops*:"() -> (w462:dbl)
        n210 = local read "Ramp (s):"() -> (w470:dbl)
        n211 = local read "New: STS"() -> (w446:dbl)
        n212 = local read "Rec: On/Off"() -> (w450:dbl)
        n213 = local read "Rec: Method"() -> (w445:string)
        n214 = local read "Date Recorded"() -> (w441:string)
        n215 = local read "Rec: Solvent"() -> (w420:string)
        n216 = local read "Time (s):"() -> (w457:dbl)
        n217 = local read "New: VT"() -> (w448:dbl)
        n218 = local read "RPM:"() -> (w458:dbl)
        n219 = local read "Fabricator:"() -> (w466:string)
        n220 = Number To Decimal String(number=w462) -> (decimal integer string=w463:string)  [unwired: 1 in]
        n221 = Number To Decimal String(number=w444) -> (decimal integer string=w437:string)  [unwired: 1 in]
        n222 = call "DeviceID"("Sample"=w437, "Year"=w438, "Month"=w432, "Day"=w428, "Index"=w426) -> ("Result"=w443:string)  [unwired: 9 in, 1 out]
        n223 = Number To Decimal String(number=w425) -> (decimal integer string=w423:string)  [unwired: 1 in]
        n224 = Number To Decimal String(number=w424) -> (decimal integer string=w422:string)  [unwired: 1 in]
        n225 = Number To Decimal String(number=w461) -> (decimal integer string=w460:string)  [unwired: 1 in]
        n226 = property on="Image Out" class="ImageControl"() -> ("ZoomSingle"=w521:cluster{"X":sgl, "Y":sgl})  [unwired: 2 in, 2 out]
        n227 = Number To Decimal String(number=w416) -> (decimal integer string=w415:string)  [unwired: 1 in]
        n228 = Number To Decimal String(number=w465) -> (decimal integer string=w464:string)  [unwired: 1 in]
        n229 = Number To Decimal String(number=w419) -> (decimal integer string=w417:string)  [unwired: 1 in]
        n230 = property on="Image Out" class="ImageControl"() -> ("Bounds"=w522:T10)  [unwired: 2 in, 2 out]
        n231 = Number To Decimal String(number=w458) -> (decimal integer string=w459:string)  [unwired: 1 in]
        n232 = Number To Fractional String(number=w452) -> (F-format string=w453:string)  [unwired: 3 in]
        n233 = Number To Decimal String(number=w457) -> (decimal integer string=w456:string)  [unwired: 1 in]
        n234 = Number To Fractional String(number=w454) -> (F-format string=w455:string)  [unwired: 3 in]
        n235 = Number To Fractional String(number=w450) -> (F-format string=w451:string)  [unwired: 3 in]
        n236 = Number To Fractional String(number=w448) -> (F-format string=w449:string)  [unwired: 3 in]
        n237 = Number To Fractional String(number=w446) -> (F-format string=w447:string)  [unwired: 3 in]
        n238 = Number To Decimal String(number=w470) -> (decimal integer string=w471:string)  [unwired: 1 in]
        n239 = call <vilib>:"Intialize Keyboard.vi"() -> ("device ID"=w533:refnum<k1>)  [unwired: 10 in, 1 out]
        n240 = property on="Image Out" class="ImageControl"() -> ("Image Center Position"=w528:cluster{"X":u32, "Y":u32})  [unwired: 2 in, 2 out]
        n241 = call-poly <vilib>:"Acquire Input Data.vi"("device ID"=w533) -> ("keys pressed"=w532:T11)  [unwired: 16 in, 2 out]
        n242 = Unbundle(w522) -> ("Width"=w519:u32, "Height"=w518:u32)
        n243 = Unbundle(w521) -> ("X"=w496:sgl, "Y"=w520:sgl)
        n244 = event shown="[3] \"Zoom\": Value Change" {
          selector: _ -> [_ _ _ _ _ _ _]
          dyn-events: _ -> [_ _ _ _ _ _ _]
          timeout: 10 -> [_ _ _ _ _ _ _]
          event "Remove Button": Mouse Down {
            w566 = 0
            n245 = property on="Image Out" class="ImageControl"() -> ("ROI"=w564:T9)  [unwired: 2 in, 2 out]
            n246 = event-data() -> ()  [unwired: 1 in, 7 out]
            n247 = Unbundle(w564) -> ("Global Rectangle"=w567:i32[], "Contours"=w569:T12)
            n248 = Reverse 1D Array(array=w567) -> (reversed array=w568:i32[])
            n249 = Reverse 1D Array(array=w569) -> (reversed array=w570:T12)
            n250 = Delete From Array(array=w568, index=w566) -> (array with subset deleted=w571:i32[])  [unwired: 1 in, 1 out]
            n251 = Delete From Array(array=w570, index=w566) -> (array with subset deleted=w572:T12)  [unwired: 1 in, 1 out]
            n252 = Reverse 1D Array(array=w571) -> (reversed array=w573:i32[])
            n253 = Reverse 1D Array(array=w572) -> (reversed array=w574:T12)
            n254 = Bundle(w573, w574) -> (w565:T13)  [unwired: 1 in]
            n255 = local write "ROI Descriptor out"(w564) -> ()
            n256 = local write "ROI Descriptor"(w565) -> ()
            n257 = property on="Image Out" class="ImageControl"("ROI"=w565) -> ()  [unwired: 2 in, 2 out]
          }
          event "Undo Button": Mouse Down {
            n258 = event-data() -> ()  [unwired: 1 in, 7 out]
            n259 = invoke on="Image Out" class="ImageControl" method="Clear ROI"() -> ()  [unwired: 3 in, 3 out]
          }
          event "Image Folder": Value Change {
            n260 = event-data() -> ()  [unwired: 1 in, 5 out]
            n261 = local read "Image File"() -> (w576:path)
            n262 = call "Vision Acquisition"("Image Path"=w576) -> ("Image Out"=w575:T2)  [unwired: 25 in, 1 out]
            n263 = local write "Image Out 2"(w575) -> ()
            n264 = local write "Image Out"(w575) -> ()
            n265 = invoke on="Image Out" class="ImageControl" method="Clear ROI"() -> ()  [unwired: 3 in, 3 out]
          }
          event "Zoom": Value Change {
            n266 = event-data() -> ()  [unwired: 1 in, 5 out]
            n267 = local read "Zoom"() -> (w577:i16)
            n268 = Bundle("Zoom"=w577, "Zoom"=w577) -> (w578:cluster{"Zoom":i16, "Zoom":i16})  [unwired: 1 in]
            n269 = property on="Image Out" class="ImageControl"("ZoomInteger"=w578) -> ()  [unwired: 2 in, 2 out]
          }
          event Timeout {
            n270 = event-data() -> ()  [unwired: 1 in, 2 out]
          }
          event "Image Out": Mouse Enter {
            (unwired) 6
            n271 = event-data() -> ()  [unwired: 1 in, 3 out]
            n272 = call "Simulate_Keyboard.vi"("Action"=0, "Virtual Key"=162) -> ()  [unwired: 7 in, 1 out]
          }
          event "Image Out": Mouse Leave {
            n273 = event-data() -> ()  [unwired: 1 in, 3 out]
            n274 = flat-sequence {
              frame #0 {
                n275 = Wait (ms)(milliseconds to wait=10) -> ()  [unwired: 1 out]
              }
              frame #1 {
                (unwired) 6
                n276 = call "Simulate_Keyboard.vi"("Action"=2, "Virtual Key"=162) -> ()  [unwired: 7 in, 1 out]
              }
            }
          }
        }
        n277 = Index Array(array=w532) -> (element=w536:T14)  [unwired: 1 in]
        n278 = Divide(x=w519, y=w496) -> (x/y=w509:sgl)
        n279 = Multiply(x=w509, y=0.5) -> (x*y=w515:dbl)
        n280 = Divide(x=w518, y=w520) -> (x/y=w508:sgl)
        n281 = Multiply(x=w508, y=0.5) -> (x*y=w514:dbl)
        n282 = Unbundle(w528) -> ("X"=w510:u32, "Y"=w511:u32)
        n283 = Subtract(x=w511, y=w514) -> (x-y=w512:dbl)
        n284 = Subtract(x=w510, y=w515) -> (x-y=w513:dbl)
        n285 = Add(x=w513, y=w509) -> (x+y=w527:dbl)
        n286 = Add(x=w512, y=w508) -> (x+y=w526:dbl)
        n287 = Build Array(w443, w466, w445, w441, w437, w467, w468, w423, w422, w414, w418, w417, w420, w421, w460, w463, w473, w464, w415, w471, w459, w453, w456, w455, w451, w449, w447) -> (w469:string[])
        n288 = local write "Current \nRecord"(w469) -> ()
        n289 = event shown="[1] \"Down Button\": Mouse Down" {
          selector: _ -> [_ _ _ _ _ _ _ _ _ _ _ _ _ _ _ _]
          dyn-events: _ -> [_ _ _ _ _ _ _ _ _ _ _ _ _ _ _ _]
          timeout: 10 -> [_ _ _ _ _ _ _ _ _ _ _ _ _ _ _ _]
          tunnel: [_ _ _ _ _ _ _ _ _ _ _ _ _ TRUE _ TRUE] -> w553
          event Timeout {
            n290 = event-data() -> ()  [unwired: 1 in, 2 out]
          }
          event "Down Button": Mouse Down {
            w910 = 0
            n291 = event-data() -> ()  [unwired: 1 in, 7 out]
            n292 = local read "NumPts 2"() -> (w871:dbl)
            n293 = local read "NumPts"() -> (w878:dbl)
            n294 = local read "Row Start"() -> (w877:dbl)
            n295 = local read "Folder Index"() -> (w835:dbl)
            n296 = local read "Data File"() -> (w915:path)
            n297 = property on="Image Out" class="ImageControl"() -> (error out=w841:errorcluster, "Image Center Position"=w845:cluster{"X":u32, "Y":u32})  [unwired: 2 in, 1 out]
            n298 = Strip Path(path=w915) -> (stripped path=w906:path, name=w927:string)
            n299 = local write "Data Folder"(w906) -> ()
            n300 = List Folder(path=w906) -> (filenames=w920:string[], error out=w850:errorcluster)  [unwired: 3 in, 2 out]
            n301 = Array Size(array=w920) -> (size(s)=w916:i32)
            n302 = Path To String(path=w906) -> (string=w928:string)
            n303 = Search 1D Array(1D array=w920, element=w927) -> (index of element=w917:i32)  [unwired: 1 in]
            n304 = Unbundle(w845) -> ("X"=w843:u32)  [unwired: 1 out]
            n305 = Unbundle() -> (w864, w863, w862, w839, w838, w837, w836)  [unwired: 1 in]
            n306 = local write "Rec: On/Off"(w862) -> ()
            n307 = Bundle("X"=w843, 0) -> (w844:cluster{"X":u32, i32})  [unwired: 1 in]
            n308 = Decrement(x=w916) -> (x-1=w918:i32)
            n309 = Equal?(x=w917, y=w918) -> (x = y?=w919:bool)
            n310 = case shown="False" w919 {
              tunnel: w835 -> [w1055 _]
              tunnel: [w1054 0] -> w834
              frame False {
                n311 = Increment(x=w1055) -> (x+1=w1054:dbl)
              }
              frame True {
              }
            }
            n312 = Index Array(array=w920, index=w834) -> (element=w921:string)
            n313 = local write "Folder Index"(w834) -> ()
            n314 = local write "Data Name"(w921) -> ()
            n315 = Concatenate Strings(w928, "\\", w921) -> (w926:string)
            n316 = property on="Image Out" class="ImageControl"(error in=w841, "Image Center Position"=w844) -> ()  [unwired: 1 in, 2 out]
            n317 = String To Path(string=w926) -> (path=w879:path)
            n318 = call "sub_thresh_swing_subvi.vi"("Path"=w879, "NumPts"=w871, "Row Start"=w877) -> ("Index"=w872:dbl, "XY Graph"=w867:cluster{dbl[], dbl[]}[], "Sub Threshold Swing"=w880:dbl)  [unwired: 8 in, 2 out]
            n319 = Decimate 1D Array(w867) -> (w870:cluster{dbl[], dbl[]}[])  [unwired: 1 out]
            n320 = Array To Cluster(array=w870) -> (cluster=w868:T8)
            n321 = Unbundle(w868) -> ("[0]"=w869:cluster{dbl[], dbl[]})  [unwired: 8 out]
            n322 = Unbundle(w869) -> (w866:dbl[], w865:dbl[])
            n323 = local write "Calc: STS"(w880) -> ()
            n324 = local write "XY Graph 2"(w867) -> ()
            n325 = local write "Index 2"(w872) -> ()
            n326 = call "mobility_subvi_07_12a_JW.vi"("Path"=w879, "NumPts"=w878, 11:w877) -> ("Dielectric (d)"=w882:dbl, "Capacitance (C)"=w840:dbl, "Index"=w887:dbl, "XY Graph"=w890:cluster{dbl[], dbl[]}[], "Length"=w881:dbl, "Vt"=w883:dbl, "Width"=w856:dbl, "Table Control"=w924:string[][], "Table Control 2"=w923:string[][], "Mobility"=w922:dbl)  [unwired: 3 in]
            n327 = local write "Rec: Dielectric (d)"(w882) -> ()
            n328 = local write "Calc: VT"(w883) -> ()
            n329 = local write "New: Dielectric"(w882) -> ()
            n330 = Decimate 1D Array(w890) -> (w891:cluster{dbl[], dbl[]}[])  [unwired: 1 out]
            n331 = Array To Cluster(array=w891) -> (cluster=w893:T8)
            n332 = local write "Table Control"(w924) -> ()
            n333 = Unbundle(w893) -> ("[0]"=w892:cluster{dbl[], dbl[]})  [unwired: 8 out]
            n334 = Unbundle(w892) -> (w874:dbl[], w873:dbl[])
            n335 = local write "Calc: Mobility-Sat"(w922) -> ()
            n336 = local write "XY Graph"(w890) -> ()
            n337 = local write "Table Control 2"(w923) -> ()
            n338 = Array Subset(array=w874, index=w887, length=w878) -> (w889:dbl[])
            n339 = Array Subset(array=w873, index=w887, length=w878) -> (w888:dbl[])
            n340 = local write "Rec: Width"(w856) -> ()
            n341 = local write "Rec: Length"(w881) -> ()
            n342 = local write "Array 2"(w888) -> ()
            n343 = local write "Array"(w889) -> ()
            n344 = local write "Device Index"(w887) -> ()
            n345 = local write "Slide"(w887) -> ()
            n346 = local write "Date Recorded"(w840) -> ()
            n347 = local write "Rec: STS"(w863) -> ()
            n348 = local write "Rec: VT"(w864) -> ()
            n349 = Array Subset(array=w866, index=w872, length=w871) -> (w876:dbl[])
            n350 = Array Subset(array=w865, index=w872, length=w871) -> (w875:dbl[])
            n351 = local write "Rec: Solvent"(w838) -> ()
            n352 = local write "Rec: Concentration"(w837) -> ()
            n353 = local write "New: Width"(w856) -> ()
            n354 = local write "Rec: Method"(w839) -> ()
            n355 = local write "Data File"(w879) -> ()
            n356 = local write "Rec: Material"(w836) -> ()
            n357 = local write "New: Length"(w881) -> ()
            n358 = local write "Array 8"(w876) -> ()
            n359 = local write "Array 7"(w875) -> ()
            n360 = call-poly <vilib>:"Read From Spreadsheet File.vi"("file path (dialog if empty)"=w879) -> ("all rows"=w912:string[][])  [unwired: 6 in, 4 out]
            n361 = local read "Image Folder"() -> (w847:path)
            n362 = Array Size(array=w912) -> (size(s)=w911:i32[])
            n363 = List Folder(path=w847, error in=w850) -> (filenames=w905:string[], error out=w851:errorcluster)  [unwired: 2 in, 2 out]
            n364 = Index Array(array=w911, index=w910) -> (element=w885:i32)
            n365 = Subtract(x=w885, y=20) -> (x-y=w884:i32)
            n366 = property on="Slide" class="Slide (strict)"("Scale.Maximum"=w884) -> ()  [unwired: 2 in, 2 out]
            n367 = Array Subset(array=w912, index (row)=w910, index (col)=w910, length (col)=3) -> (w913:string[][])  [unwired: 1 in]
            n368 = Reshape Array(w913, w885) -> (w894:string[])
            n369 = local read "No Image"() -> (w857:path)
            n370 = Search 1D Array(1D array=w894, element="Mobility-Sat (cm^2/Vs):") -> (index of element=w899:i32)  [unwired: 1 in]
            n371 = Search 1D Array(1D array=w894, element="Index:") -> (index of element=w907:i32)  [unwired: 1 in]
            n372 = Increment(x=w907) -> (x+1=w908:i32)
            n373 = Index Array(array=w894, index=w908) -> (element=w849:string)
            n374 = while {
              tunnel: w905 -> [w941]
              tunnel: w849 -> [w939]
              tunnel: [w938] -> _
              tunnel: [w938] -> w904
              tunnel: w885 -> [w937]
              i -> [w938]
              stop <- w934 stop-if-true
              n375 = Index Array(array=w941, index=w938) -> (element=w942:string)
              n376 = xnode "Match Regular Expression"("input string"=w942, "regular expression"=w939) -> ("whole match"=w940:string)  [unwired: 4 in, 4 out]
              n377 = Equal?(x=w940, y=w939) -> (x = y?=w936:bool)
              n378 = Equal?(x=w937, y=w938) -> (x = y?=w935:bool)
              n379 = Or(x=w936, y=w935) -> (x .or. y?=w934:bool)
            }
            n380 = local write "Index"(w849) -> ()
            n381 = Increment(x=w899) -> (x+1=w898:i32)
            n382 = Build Path(base path=w847, name or relative path="ROI") -> (appended path=w846:path)
            n383 = Index Array(array=w894, index=w898) -> (element=w896:string)
            n384 = Fract/Exp String To Number(string=w896) -> (number=w895:dbl)  [unwired: 3 in, 1 out]
            n385 = local write "Rec: Mobility-Sat"(w895) -> ()
            n386 = Build Path(base path=w846, name or relative path=w849) -> (appended path=w855:path)
            n387 = invoke on="Image Out" class="ImageControl" method="Clear ROI"(error in=w851) -> (error out=w854:errorcluster)  [unwired: 2 in, 2 out]
            n388 = Path To String(path=w847) -> (string=w902:string)
            n389 = call <vilib>:"Check if File or Folder Exists.vi"("error in (no error)"=w854, "path"=w855) -> ("file or folder exists?"=w852:bool, "dup path"=w853:path)  [unwired: 7 in, 1 out]
            n390 = case shown="True" w852 {
              tunnel: w853 -> [_ w929]
              frame False {
              }
              frame True {
                n391 = Read from Text File(file (use dialog)=w929) -> (text=w933:string)  [unwired: 3 in, 3 out]
                n392 = property on="Image Out" class="ImageControl"() -> ("ROI"=w930:T9)  [unwired: 2 in, 2 out]
                n393 = Unflatten From String(type=w930, binary string=w933) -> (value=w931:T9, error out=w932:errorcluster)  [unwired: 3 in, 1 out]
                n394 = property on="Image Out" class="ImageControl"(error in=w932, "ROI"=w931) -> ()  [unwired: 1 in, 2 out]
              }
            }
            n395 = Index Array(array=w905, index=w904) -> (element=w860:string)
            n396 = Empty String/Path?(string/path=w860) -> (empty?=w861:bool)
            n397 = Concatenate Strings(w902, "\\", w860) -> (w901:string)
            n398 = String To Path(string=w901) -> (path=w859:path)
            n399 = Select(t=w857, s=w861, f=w859) -> (s? t:f=w858:path)
            n400 = call "Vision Acquisition4"("Image Path"=w858) -> ("Image Out"=w903:T2)  [unwired: 25 in, 1 out]
            n401 = local write "Image File"(w858) -> ()
            n402 = local write "Image Out 2"(w903) -> ()
            n403 = local write "Image Out"(w903) -> ()
            n404 = invoke on="Image Out" class="ImageControl" method="Clear ROI"() -> ()  [unwired: 3 in, 3 out]
            n405 = local write "Image Name"(w860) -> ()
          }
          event "Data File": Value Change {
            w1128 = 0
            n406 = event-data() -> ()  [unwired: 1 in, 5 out]
            n407 = local read "NumPts"() -> (w1096:dbl)
            n408 = local read "Row Start"() -> (w1095:dbl)
            n409 = local read "Data File"() -> (w1124:path)
            n410 = local read "NumPts 2"() -> (w1089:dbl)
            n411 = property on="Image Out" class="ImageControl"() -> (error out=w1058:errorcluster, "Image Center Position"=w1062:cluster{"X":u32, "Y":u32})  [unwired: 2 in, 1 out]
            n412 = Strip Path(path=w1124) -> (stripped path=w1123:path, name=w1140:string)
            n413 = local write "Data Folder"(w1123) -> ()
            n414 = List Folder(path=w1123) -> (filenames=w1133:string[], error out=w1068:errorcluster)  [unwired: 3 in, 2 out]
            n415 = Unbundle(w1062) -> ("X"=w1060:u32)  [unwired: 1 out]
            n416 = Path To String(path=w1123) -> (string=w1141:string)
            n417 = Search 1D Array(1D array=w1133, element=w1140) -> (index of element=w1057:i32)  [unwired: 1 in]
            n418 = Index Array(array=w1133, index=w1057) -> (element=w1134:string)
            n419 = Bundle("X"=w1060, 0) -> (w1061:cluster{"X":u32, i32})  [unwired: 1 in]
            n420 = Unbundle() -> ("Vt"=w1081, "STS"=w1080, "On/Off"=w1079)  [unwired: 1 in]
            n421 = local write "Rec: On/Off"(w1079) -> ()
            n422 = local write "Data Name"(w1134) -> ()
            n423 = property on="Image Out" class="ImageControl"(error in=w1058, "Image Center Position"=w1061) -> ()  [unwired: 1 in, 2 out]
            n424 = local write "Folder Index"(w1057) -> ()
            n425 = Concatenate Strings(w1141, "\\", w1134) -> (w1139:string)
            n426 = local write "Rec: STS"(w1080) -> ()
            n427 = local write "Rec: VT"(w1081) -> ()
            n428 = String To Path(string=w1139) -> (path=w1097:path)
            n429 = call "sub_thresh_swing_subvi.vi"("Path"=w1097, "NumPts"=w1089, "Row Start"=w1095) -> ("Index"=w1090:dbl, "XY Graph"=w1085:cluster{dbl[], dbl[]}[], "Sub Threshold Swing"=w1094:dbl)  [unwired: 8 in, 2 out]
            n430 = Decimate 1D Array(w1085) -> (w1088:cluster{dbl[], dbl[]}[])  [unwired: 1 out]
            n431 = Array To Cluster(array=w1088) -> (cluster=w1086:T8)
            n432 = Unbundle(w1086) -> ("[0]"=w1087:cluster{dbl[], dbl[]})  [unwired: 8 out]
            n433 = Unbundle(w1087) -> (w1083:dbl[], w1082:dbl[])
            n434 = local write "Index 2"(w1090) -> ()
            n435 = call "mobility_subvi_07_12a_JW.vi"("Path"=w1097, "NumPts"=w1096, 11:w1095) -> ("Dielectric (d)"=w1099:dbl, "Index"=w1104:dbl, "XY Graph"=w1107:cluster{dbl[], dbl[]}[], "Length"=w1098:dbl, "Vt"=w1100:dbl, "Width"=w1073:dbl, "Table Control"=w1137:string[][], "Table Control 2"=w1136:string[][], "Mobility"=w1135:dbl)  [unwired: 3 in, 1 out]
            n436 = local write "Rec: Dielectric (d)"(w1099) -> ()
            n437 = local write "New: Dielectric"(w1099) -> ()
            n438 = Decimate 1D Array(w1107) -> (w1108:cluster{dbl[], dbl[]}[])  [unwired: 1 out]
            n439 = local write "Table Control"(w1137) -> ()
            n440 = Array To Cluster(array=w1108) -> (cluster=w1110:T8)
            n441 = Unbundle(w1110) -> ("[0]"=w1109:cluster{dbl[], dbl[]})  [unwired: 8 out]
            n442 = local write "Calc: VT"(w1100) -> ()
            n443 = local write "Calc: STS"(w1094) -> ()
            n444 = local write "Calc: Mobility-Sat"(w1135) -> ()
            n445 = Unbundle(w1109) -> (w1084:dbl[], w1091:dbl[])
            n446 = local write "XY Graph"(w1107) -> ()
            n447 = local write "Rec: Length"(w1098) -> ()
            n448 = local write "Table Control 2"(w1136) -> ()
            n449 = local write "XY Graph 2"(w1085) -> ()
            n450 = Array Subset(array=w1083, index=w1090, length=w1089) -> (w1093:dbl[])
            n451 = Array Subset(array=w1082, index=w1090, length=w1089) -> (w1092:dbl[])
            n452 = local write "Rec: Width"(w1073) -> ()
            n453 = Array Subset(array=w1084, index=w1104, length=w1096) -> (w1106:dbl[])
            n454 = Array Subset(array=w1091, index=w1104, length=w1096) -> (w1105:dbl[])
            n455 = local write "Array 8"(w1093) -> ()
            n456 = local write "Array 7"(w1092) -> ()
            n457 = local write "New: Length"(w1098) -> ()
            n458 = local write "New: Width"(w1073) -> ()
            n459 = local write "Array 2"(w1105) -> ()
            n460 = local write "Array"(w1106) -> ()
            n461 = local write "Data File"(w1097) -> ()
            n462 = local write "Device Index"(w1104) -> ()
            n463 = local read "Image Folder"() -> (w1064:path)
            n464 = local write "Slide"(w1104) -> ()
            n465 = List Folder(path=w1064, error in=w1068) -> (filenames=w1121:string[], error out=w1067:errorcluster)  [unwired: 2 in, 2 out]
            n466 = call-poly <vilib>:"Read From Spreadsheet File.vi"("file path (dialog if empty)"=w1097) -> ("all rows"=w1130:string[][])  [unwired: 6 in, 4 out]
            n467 = Array Size(array=w1130) -> (size(s)=w1129:i32[])
            n468 = Index Array(array=w1129, index=w1128) -> (element=w1103:i32)
            n469 = Subtract(x=w1103, y=20) -> (x-y=w1101:i32)
            n470 = property on="Slide" class="Slide (strict)"("Scale.Maximum"=w1101) -> ()  [unwired: 2 in, 2 out]
            n471 = Array Subset(array=w1130, index (row)=w1128, index (col)=w1128, length (col)=3) -> (w1131:string[][])  [unwired: 1 in]
            n472 = Reshape Array(w1131, w1103) -> (w1111:string[])
            n473 = Search 1D Array(1D array=w1111, element="Index:") -> (index of element=w1125:i32)  [unwired: 1 in]
            n474 = Increment(x=w1125) -> (x+1=w1126:i32)
            n475 = Index Array(array=w1111, index=w1126) -> (element=w1066:string)
            n476 = while {
              tunnel: w1121 -> [w1154]
              tunnel: w1066 -> [w1152]
              tunnel: [w1151] -> _
              tunnel: [w1151] -> w1120
              tunnel: w1103 -> [w1150]
              i -> [w1151]
              stop <- w1147 stop-if-true
              n477 = Index Array(array=w1154, index=w1151) -> (element=w1155:string)
              n478 = xnode "Match Regular Expression"("input string"=w1155, "regular expression"=w1152) -> ("whole match"=w1153:string)  [unwired: 4 in, 4 out]
              n479 = Equal?(x=w1153, y=w1152) -> (x = y?=w1149:bool)
              n480 = Equal?(x=w1150, y=w1151) -> (x = y?=w1148:bool)
              n481 = Or(x=w1149, y=w1148) -> (x .or. y?=w1147:bool)
            }
            n482 = local write "Index"(w1066) -> ()
            n483 = Search 1D Array(1D array=w1111, element="Mobility-Sat (cm^2/Vs):") -> (index of element=w1116:i32)  [unwired: 1 in]
            n484 = Increment(x=w1116) -> (x+1=w1115:i32)
            n485 = Index Array(array=w1111, index=w1115) -> (element=w1113:string)
            n486 = Fract/Exp String To Number(string=w1113) -> (number=w1112:dbl)  [unwired: 3 in, 1 out]
            n487 = local write "Rec: Mobility-Sat"(w1112) -> ()
            n488 = Build Path(base path=w1064, name or relative path="ROI") -> (appended path=w1063:path)
            n489 = Path To String(path=w1064) -> (string=w1119:string)
            n490 = local read "No Image"() -> (w1074:path)
            n491 = Build Path(base path=w1063, name or relative path=w1066) -> (appended path=w1072:path)
            n492 = invoke on="Image Out" class="ImageControl" method="Clear ROI"(error in=w1067) -> (error out=w1071:errorcluster)  [unwired: 2 in, 2 out]
            n493 = Index Array(array=w1121, index=w1120) -> (element=w1077:string)
            n494 = Empty String/Path?(string/path=w1077) -> (empty?=w1078:bool)
            n495 = Concatenate Strings(w1119, "\\", w1077) -> (w1118:string)
            n496 = String To Path(string=w1118) -> (path=w1076:path)
            n497 = Select(t=w1074, s=w1078, f=w1076) -> (s? t:f=w1075:path)
            n498 = call "Vision Acquisition3"("Image Path"=w1075) -> ("Image Out"=w1122:T2)  [unwired: 25 in, 1 out]
            n499 = local write "Image File"(w1075) -> ()
            n500 = local write "Image Out 2"(w1122) -> ()
            n501 = local write "Image Out"(w1122) -> ()
            n502 = local write "Image Name"(w1077) -> ()
            n503 = call <vilib>:"Check if File or Folder Exists.vi"("error in (no error)"=w1071, "path"=w1072) -> ("file or folder exists?"=w1069:bool, "dup path"=w1070:path)  [unwired: 7 in, 1 out]
            n504 = invoke on="Image Out" class="ImageControl" method="Clear ROI"() -> ()  [unwired: 3 in, 3 out]
            n505 = case shown="True" w1069 {
              tunnel: w1070 -> [_ w1142]
              frame False {
              }
              frame True {
                n506 = Read from Text File(file (use dialog)=w1142) -> (text=w1146:string)  [unwired: 3 in, 3 out]
                n507 = property on="Image Out" class="ImageControl"() -> ("ROI"=w1143:T9)  [unwired: 2 in, 2 out]
                n508 = Unflatten From String(type=w1143, binary string=w1146) -> (value=w1144:T9, error out=w1145:errorcluster)  [unwired: 3 in, 1 out]
                n509 = property on="Image Out" class="ImageControl"(error in=w1145, "ROI"=w1144) -> ()  [unwired: 1 in, 2 out]
              }
            }
          }
          event "Up Button": Mouse Down {
            w1341 = 0
            n510 = event-data() -> ()  [unwired: 1 in, 5 out]
            n511 = local read "Folder Index"() -> (w1268:dbl)
            n512 = local read "Row Start"() -> (w1311:dbl)
            n513 = local read "Data File"() -> (w1337:path)
            n514 = local read "NumPts 2"() -> (w1306:dbl)
            n515 = local read "NumPts"() -> (w1312:dbl)
            n516 = property on="Image Out" class="ImageControl"() -> (error out=w1272:errorcluster, "Image Center Position"=w1276:cluster{"X":u32, "Y":u32})  [unwired: 2 in, 1 out]
            n517 = Strip Path(path=w1337) -> (stripped path=w1336:path, name=w1355:string)
            n518 = local write "Data Folder"(w1336) -> ()
            n519 = List Folder(path=w1336) -> (filenames=w1346:string[], error out=w1282:errorcluster)  [unwired: 3 in, 2 out]
            n520 = Path To String(path=w1336) -> (string=w1356:string)
            n521 = Search 1D Array(1D array=w1346, element=w1355) -> (index of element=w1347:i32)  [unwired: 1 in]
            n522 = Unbundle(w1276) -> ("X"=w1274:u32)  [unwired: 1 out]
            n523 = Equal To 0?(x=w1347) -> (x = 0?=w1348:bool)
            n524 = Bundle("X"=w1274, 0) -> (w1275:cluster{"X":u32, i32})  [unwired: 1 in]
            n525 = property on="Image Out" class="ImageControl"(error in=w1272, "Image Center Position"=w1275) -> ()  [unwired: 1 in, 2 out]
            n526 = Unbundle() -> ("Vt"=w1298, "STS"=w1297, "On/Off"=w1296)  [unwired: 1 in]
            n527 = Array Size(array=w1346) -> (size(s)=w1269:i32)
            n528 = case shown="True" w1348 {
              tunnel: w1268 -> [w1483 _]
              tunnel: [w1482 w1484] -> w1267
              tunnel: w1269 -> [_ w1485]
              frame False {
                n529 = Decrement(x=w1483) -> (x-1=w1482:dbl)
              }
              frame True {
                n530 = Decrement(x=w1485) -> (x-1=w1484:i32)
              }
            }
            n531 = Index Array(array=w1346, index=w1267) -> (element=w1349:string)
            n532 = local write "Data Name"(w1349) -> ()
            n533 = local write "Folder Index"(w1267) -> ()
            n534 = Concatenate Strings(w1356, "\\", w1349) -> (w1354:string)
            n535 = String To Path(string=w1354) -> (path=w1313:path)
            n536 = call "sub_thresh_swing_subvi.vi"("Path"=w1313, "NumPts"=w1306, "Row Start"=w1311) -> ("Index"=w1305:dbl, "XY Graph"=w1301:cluster{dbl[], dbl[]}[], "Sub Threshold Swing"=w1314:dbl)  [unwired: 8 in, 2 out]
            n537 = Decimate 1D Array(w1301) -> (w1304:cluster{dbl[], dbl[]}[])  [unwired: 1 out]
            n538 = Array To Cluster(array=w1304) -> (cluster=w1302:T8)
            n539 = Unbundle(w1302) -> ("[0]"=w1303:cluster{dbl[], dbl[]})  [unwired: 8 out]
            n540 = Unbundle(w1303) -> (w1300:dbl[], w1299:dbl[])
            n541 = Array Subset(array=w1299, index=w1305, length=w1306) -> (w1307:dbl[])
            n542 = Array Subset(array=w1300, index=w1305, length=w1306) -> (w1308:dbl[])
            n543 = local write "Calc: STS"(w1314) -> ()
            n544 = local write "Array 8"(w1308) -> ()
            n545 = local write "Array 7"(w1307) -> ()
            n546 = call "mobility_subvi_07_12a_JW.vi"("Path"=w1313, "NumPts"=w1312, 11:w1311) -> ("Dielectric (d)"=w1316:dbl, "Capacitance (C)"=w1271:dbl, "Index"=w1318:dbl, "XY Graph"=w1324:cluster{dbl[], dbl[]}[], "Length"=w1315:dbl, "Vt"=w1317:dbl, "Width"=w1293:dbl, "Table Control"=w1352:string[][], "Table Control 2"=w1351:string[][], "Mobility"=w1350:dbl)  [unwired: 3 in]
            n547 = local write "Rec: Dielectric (d)"(w1316) -> ()
            n548 = local write "New: Dielectric"(w1316) -> ()
            n549 = local write "New: Length"(w1315) -> ()
            n550 = local write "New: Width"(w1293) -> ()
            n551 = local write "Table Control"(w1352) -> ()
            n552 = Decimate 1D Array(w1324) -> (w1325:cluster{dbl[], dbl[]}[])  [unwired: 1 out]
            n553 = local write "XY Graph 2"(w1301) -> ()
            n554 = local write "Calc: Mobility-Sat"(w1350) -> ()
            n555 = Array To Cluster(array=w1325) -> (cluster=w1327:T8)
            n556 = local write "XY Graph"(w1324) -> ()
            n557 = local write "Rec: Length"(w1315) -> ()
            n558 = local write "Index 2"(w1305) -> ()
            n559 = local write "Table Control 2"(w1351) -> ()
            n560 = Unbundle(w1327) -> ("[0]"=w1326:cluster{dbl[], dbl[]})  [unwired: 8 out]
            n561 = local write "Date Recorded"(w1271) -> ()
            n562 = Unbundle(w1326) -> (w1310:dbl[], w1309:dbl[])
            n563 = local write "Calc: VT"(w1317) -> ()
            n564 = local write "Rec: Width"(w1293) -> ()
            n565 = local write "Device Index"(w1318) -> ()
            n566 = Array Subset(array=w1310, index=w1318, length=w1312) -> (w1323:dbl[])
            n567 = Array Subset(array=w1309, index=w1318, length=w1312) -> (w1322:dbl[])
            n568 = local write "Data File"(w1313) -> ()
            n569 = local write "Rec: STS"(w1297) -> ()
            n570 = local write "Rec: VT"(w1298) -> ()
            n571 = local write "Rec: On/Off"(w1296) -> ()
            n572 = local write "Array 2"(w1322) -> ()
            n573 = local write "Array"(w1323) -> ()
            n574 = local read "Image Folder"() -> (w1270:path)
            n575 = local write "Slide"(w1318) -> ()
            n576 = List Folder(path=w1270, error in=w1282) -> (filenames=w1335:string[], error out=w1281:errorcluster)  [unwired: 2 in, 2 out]
            n577 = call-poly <vilib>:"Read From Spreadsheet File.vi"("file path (dialog if empty)"=w1313) -> ("all rows"=w1343:string[][])  [unwired: 6 in, 4 out]
            n578 = Array Size(array=w1343) -> (size(s)=w1342:i32[])
            n579 = Index Array(array=w1342, index=w1341) -> (element=w1320:i32)
            n580 = Subtract(x=w1320, y=20) -> (x-y=w1319:i32)
            n581 = property on="Slide" class="Slide (strict)"("Scale.Maximum"=w1319) -> ()  [unwired: 2 in, 2 out]
            n582 = Array Subset(array=w1343, index (row)=w1341, index (col)=w1341, length (col)=3) -> (w1344:string[][])  [unwired: 1 in]
            n583 = Reshape Array(w1344, w1320) -> (w1330:string[])
            n584 = Search 1D Array(1D array=w1330, element="Mobility-Sat (cm^2/Vs):") -> (index of element=w1333:i32)  [unwired: 1 in]
            n585 = Increment(x=w1333) -> (x+1=w1332:i32)
            n586 = Index Array(array=w1330, index=w1332) -> (element=w1329:string)
            n587 = Fract/Exp String To Number(string=w1329) -> (number=w1328:dbl)  [unwired: 3 in, 1 out]
            n588 = local write "Rec: Mobility-Sat"(w1328) -> ()
            n589 = Search 1D Array(1D array=w1330, element="Index:") -> (index of element=w1338:i32)  [unwired: 1 in]
            n590 = Increment(x=w1338) -> (x+1=w1339:i32)
            n591 = Index Array(array=w1330, index=w1339) -> (element=w1278:string)
            n592 = while {
              tunnel: w1335 -> [w1369]
              tunnel: w1278 -> [w1367]
              tunnel: [w1366] -> w1334
              tunnel: w1320 -> [w1365]
              i -> [w1366]
              stop <- w1362 stop-if-true
              n593 = Index Array(array=w1369, index=w1366) -> (element=w1370:string)
              n594 = xnode "Match Regular Expression"("input string"=w1370, "regular expression"=w1367) -> ("whole match"=w1368:string)  [unwired: 4 in, 4 out]
              n595 = Equal?(x=w1368, y=w1367) -> (x = y?=w1364:bool)
              n596 = Equal?(x=w1365, y=w1366) -> (x = y?=w1363:bool)
              n597 = Or(x=w1364, y=w1363) -> (x .or. y?=w1362:bool)
            }
            n598 = local write "Index"(w1278) -> ()
            n599 = Build Path(base path=w1270, name or relative path="ROI") -> (appended path=w1279:path)
            n600 = Build Path(base path=w1279, name or relative path=w1278) -> (appended path=w1277:path)
            n601 = invoke on="Image Out" class="ImageControl" method="Clear ROI"(error in=w1281) -> (error out=w1285:errorcluster)  [unwired: 2 in, 2 out]
            n602 = call <vilib>:"Check if File or Folder Exists.vi"("error in (no error)"=w1285, "path"=w1277) -> ("file or folder exists?"=w1283:bool, "dup path"=w1284:path)  [unwired: 7 in, 1 out]
            n603 = local read "No Image"() -> (w1294:path)
            n604 = Index Array(array=w1335, index=w1334) -> (element=w1287:string)
            n605 = Build Path(base path=w1270, name or relative path=w1287) -> (appended path=w1286:path)
            n606 = local write "Image Name"(w1287) -> ()
            n607 = case shown="True" w1283 {
              tunnel: w1284 -> [_ w1357]
              frame False {
              }
              frame True {
                n608 = Read from Text File(file (use dialog)=w1357) -> (text=w1361:string)  [unwired: 3 in, 3 out]
                n609 = property on="Image Out" class="ImageControl"() -> ("ROI"=w1358:T9)  [unwired: 2 in, 2 out]
                n610 = Unflatten From String(type=w1358, binary string=w1361) -> (value=w1359:T9, error out=w1360:errorcluster)  [unwired: 3 in, 1 out]
                n611 = property on="Image Out" class="ImageControl"(error in=w1360, "ROI"=w1359) -> ()  [unwired: 1 in, 2 out]
              }
            }
            n612 = Empty String/Path?(string/path=w1287) -> (empty?=w1295:bool)
            n613 = Select(t=w1294, s=w1295, f=w1286) -> (s? t:f=w1288:path)
            n614 = call "Vision Acquisition5"("Image Path"=w1288) -> ("Image Out"=w1292:T2)  [unwired: 25 in, 1 out]
            n615 = local write "Image File"(w1288) -> ()
            n616 = local write "Image Out 2"(w1292) -> ()
            n617 = local write "Image Out"(w1292) -> ()
            n618 = call <vilib>:"Get File Extension.vi"("file"=w1288) -> ("lowercase file extension"=w1290:string)  [unwired: 7 in, 3 out]
            n619 = local write "String"(w1290) -> ()
            n620 = Search 1D Array(1D array=string[] ["bmp", "jpeg", "png", "jpg", "gif"], element=w1290) -> (index of element=w1289:i32)  [unwired: 1 in]
            n621 = Less Than 0?(x=w1289) -> ()  [unwired: 1 out]
          }
          event "Save Changes? 3": Mouse Down {
            n622 = event-data() -> ()  [unwired: 1 in, 7 out]
            n623 = local read "Image Folder"() -> (w1486:path)
            n624 = Build Path(base path=w1486, name or relative path="ROI") -> (appended path=w1493:path)
            n625 = call <vilib>:"Check if File or Folder Exists.vi"("path"=w1493) -> ("file or folder exists?"=w1495:bool, "dup path"=w1492:path)  [unwired: 8 in, 1 out]
            n626 = case shown="False" w1495 {
              tunnel: w1492 -> [w1497 w1498]
              tunnel: [w1496 w1498] -> w1487
              frame False {
                n627 = Create Folder(path (use dialog)=w1497) -> (created path=w1496:path)  [unwired: 2 in, 2 out]
              }
              frame True {
              }
            }
            n628 = property on="Image Out" class="ImageControl"() -> ("ROI"=w1491:T9)  [unwired: 2 in, 2 out]
            n629 = local read "Index"() -> (w1489:string)
            n630 = Flatten To String(anything=w1491) -> (data string=w1490:string)  [unwired: 3 in, 2 out]
            n631 = Build Path(base path=w1487, name or relative path=w1489) -> (appended path=w1488:path)
            n632 = Write to Text File(file (use dialog)=w1488, text=w1490) -> ()  [unwired: 2 in, 3 out]
          }
          event "Next Button": Mouse Down {
            n633 = event-data() -> ()  [unwired: 1 in, 5 out]
            n634 = local read "XY Graph"() -> (w1511:cluster{dbl[], dbl[]}[])
            n635 = local read "Device Index"() -> (w1513:dbl)
            n636 = local read "NumPts"() -> (w1512:dbl)
            n637 = Decimate 1D Array(w1511) -> (w1507:cluster{dbl[], dbl[]}[], w1506:cluster{dbl[], dbl[]}[])
            n638 = Array To Cluster(array=w1507) -> (cluster=w1517:T8)
            n639 = Unbundle(w1517) -> ("[0]"=w1516:cluster{dbl[], dbl[]})  [unwired: 8 out]
            n640 = Increment(x=w1513) -> (x+1=w1508:dbl)
            n641 = Unbundle(w1516) -> (w1515:dbl[], w1514:dbl[])
            n642 = local write "Device Index"(w1508) -> ()
            n643 = Array Subset(array=w1515, index=w1508, length=w1512) -> (w1504:dbl[])
            n644 = Array Subset(array=w1514, index=w1508, length=w1512) -> (w1503:dbl[])
            n645 = Bundle(w1504, w1503) -> (w1510:cluster{dbl[], dbl[]})  [unwired: 1 in]
            n646 = Build Array (concatenate)(w1507, w1506, w1510) -> (w1509:cluster{dbl[], dbl[]}[])
            n647 = local write "XY Graph"(w1509) -> ()
            n648 = local read "New: Dielectric"() -> (w1502:dbl)
            n649 = local write "Array 2"(w1503) -> ()
            n650 = local read "New: Length"() -> (w1501:dbl)
            n651 = local write "Array"(w1504) -> ()
            n652 = local read "New: Width"() -> (w1500:dbl)
            n653 = call "mob_calc_subvi.vi"("Width"=w1500, "Length"=w1501, "Dielectric (d)"=w1502, "Array 2"=w1503, "Array"=w1504) -> ("Vt"=w1499:dbl, "Mobility"=w1505:dbl)  [unwired: 4 in, 1 out]
            n654 = local write "New: Mobility-Sat"(w1505) -> ()
            n655 = local write "New: VT"(w1499) -> ()
          }
          event "Next Button 2": Mouse Down {
            n656 = event-data() -> ()  [unwired: 1 in, 7 out]
            n657 = local read "XY Graph 2"() -> (w1526:cluster{dbl[], dbl[]}[])
            n658 = local read "Index 2"() -> (w1528:dbl)
            n659 = local read "NumPts 2"() -> (w1527:dbl)
            n660 = Decimate 1D Array(w1526) -> (w1522:cluster{dbl[], dbl[]}[], w1521:cluster{dbl[], dbl[]}[])
            n661 = Array To Cluster(array=w1522) -> (cluster=w1532:T8)
            n662 = Unbundle(w1532) -> ("[0]"=w1531:cluster{dbl[], dbl[]})  [unwired: 8 out]
            n663 = Increment(x=w1528) -> (x+1=w1523:dbl)
            n664 = Unbundle(w1531) -> (w1530:dbl[], w1529:dbl[])
            n665 = local write "Index 2"(w1523) -> ()
            n666 = Array Subset(array=w1530, index=w1523, length=w1527) -> (w1519:dbl[])
            n667 = Array Subset(array=w1529, index=w1523, length=w1527) -> (w1518:dbl[])
            n668 = Bundle(w1519, w1518) -> (w1525:cluster{dbl[], dbl[]})  [unwired: 1 in]
            n669 = Build Array (concatenate)(w1522, w1521, w1525) -> (w1524:cluster{dbl[], dbl[]}[])
            n670 = local write "XY Graph 2"(w1524) -> ()
            n671 = local write "Array 8"(w1519) -> ()
            n672 = call "sts_calc_subvi.vi"("Array 2"=w1519, "Array"=w1518) -> ("STS"=w1520:dbl)  [unwired: 9 in]
            n673 = local write "Array 7"(w1518) -> ()
            n674 = local write "New: STS"(w1520) -> ()
          }
          event "Previous Button 2": Mouse Down {
            n675 = event-data() -> ()  [unwired: 1 in, 7 out]
            n676 = local read "XY Graph 2"() -> (w1542:cluster{dbl[], dbl[]}[])
            n677 = local read "NumPts 2"() -> (w1543:dbl)
            n678 = local read "Index 2"() -> (w1535:dbl)
            n679 = Decimate 1D Array(w1542) -> (w1539:cluster{dbl[], dbl[]}[], w1538:cluster{dbl[], dbl[]}[])
            n680 = Array To Cluster(array=w1539) -> (cluster=w1547:T8)
            n681 = Unbundle(w1547) -> ("[0]"=w1546:cluster{dbl[], dbl[]})  [unwired: 8 out]
            n682 = Decrement(x=w1535) -> (x-1=w1536:dbl)
            n683 = Unbundle(w1546) -> (w1545:dbl[], w1544:dbl[])
            n684 = local write "Index 2"(w1536) -> ()
            n685 = Array Subset(array=w1545, index=w1536, length=w1543) -> (w1533:dbl[])
            n686 = Array Subset(array=w1544, index=w1536, length=w1543) -> (w1534:dbl[])
            n687 = Bundle(w1533, w1534) -> (w1541:cluster{dbl[], dbl[]})  [unwired: 1 in]
            n688 = Build Array (concatenate)(w1539, w1538, w1541) -> (w1540:cluster{dbl[], dbl[]}[])
            n689 = local write "XY Graph 2"(w1540) -> ()
            n690 = local write "Array 7"(w1534) -> ()
            n691 = call "sts_calc_subvi.vi"("Array 2"=w1533, "Array"=w1534) -> ("STS"=w1537:dbl)  [unwired: 9 in]
            n692 = local write "Array 8"(w1533) -> ()
            n693 = local write "New: STS"(w1537) -> ()
          }
          event "Previous Button": Mouse Down {
            n694 = event-data() -> ()  [unwired: 1 in, 5 out]
            n695 = local read "XY Graph"() -> (w1561:cluster{dbl[], dbl[]}[])
            n696 = Decimate 1D Array(w1561) -> (w1558:cluster{dbl[], dbl[]}[], w1557:cluster{dbl[], dbl[]}[])
            n697 = local read "Device Index"() -> (w1556:dbl)
            n698 = local read "NumPts"() -> (w1562:dbl)
            n699 = Array To Cluster(array=w1558) -> (cluster=w1566:T8)
            n700 = Unbundle(w1566) -> ("[0]"=w1565:cluster{dbl[], dbl[]})  [unwired: 8 out]
            n701 = Decrement(x=w1556) -> (x-1=w1555:dbl)
            n702 = Unbundle(w1565) -> (w1564:dbl[], w1563:dbl[])
            n703 = local read "New: Dielectric"() -> (w1549:dbl)
            n704 = Array Subset(array=w1564, index=w1555, length=w1562) -> (w1554:dbl[])
            n705 = local write "Device Index"(w1555) -> ()
            n706 = Array Subset(array=w1563, index=w1555, length=w1562) -> (w1553:dbl[])
            n707 = Bundle(w1554, w1553) -> (w1560:cluster{dbl[], dbl[]})  [unwired: 1 in]
            n708 = Build Array (concatenate)(w1558, w1557, w1560) -> (w1559:cluster{dbl[], dbl[]}[])
            n709 = local write "XY Graph"(w1559) -> ()
            n710 = local read "New: Length"() -> (w1550:dbl)
            n711 = local write "Array 2"(w1553) -> ()
            n712 = local read "New: Width"() -> (w1551:dbl)
            n713 = call "mob_calc_subvi.vi"("Width"=w1551, "Length"=w1550, "Dielectric (d)"=w1549, "Array 2"=w1553, "Array"=w1554) -> ("Vt"=w1548:dbl, "Mobility"=w1552:dbl)  [unwired: 4 in, 1 out]
            n714 = local write "New: Mobility-Sat"(w1552) -> ()
            n715 = local write "Array"(w1554) -> ()
            n716 = local write "New: VT"(w1548) -> ()
          }
          event "Slide": Value Change {
            n717 = event-data() -> ()  [unwired: 1 in, 5 out]
            n718 = local read "XY Graph"() -> (w1579:cluster{dbl[], dbl[]}[])
            n719 = local read "Slide"() -> (w1568:dbl)
            n720 = Decimate 1D Array(w1579) -> (w1576:cluster{dbl[], dbl[]}[], w1575:cluster{dbl[], dbl[]}[])
            n721 = local read "NumPts"() -> (w1580:dbl)
            n722 = Array To Cluster(array=w1576) -> (cluster=w1584:T8)
            n723 = Unbundle(w1584) -> ("[0]"=w1583:cluster{dbl[], dbl[]})  [unwired: 8 out]
            n724 = Unbundle(w1583) -> (w1582:dbl[], w1581:dbl[])
            n725 = local read "New: Dielectric"() -> (w1569:dbl)
            n726 = Array Subset(array=w1582, index=w1568, length=w1580) -> (w1574:dbl[])
            n727 = local write "Device Index"(w1568) -> ()
            n728 = Array Subset(array=w1581, index=w1568, length=w1580) -> (w1573:dbl[])
            n729 = Bundle(w1574, w1573) -> (w1578:cluster{dbl[], dbl[]})  [unwired: 1 in]
            n730 = Build Array (concatenate)(w1576, w1575, w1578) -> (w1577:cluster{dbl[], dbl[]}[])
            n731 = local write "XY Graph"(w1577) -> ()
            n732 = local read "New: Length"() -> (w1570:dbl)
            n733 = local write "Array 2"(w1573) -> ()
            n734 = local read "New: Width"() -> (w1571:dbl)
            n735 = call "mob_calc_subvi.vi"("Width"=w1571, "Length"=w1570, "Dielectric (d)"=w1569, "Array 2"=w1573, "Array"=w1574) -> ("Vt"=w1567:dbl, "Mobility"=w1572:dbl)  [unwired: 4 in, 1 out]
            n736 = local write "New: Mobility-Sat"(w1572) -> ()
            n737 = local write "Array"(w1574) -> ()
            n738 = local write "New: VT"(w1567) -> ()
          }
          event "Slide 2": Value Change {
            n739 = event-data() -> ()  [unwired: 1 in, 5 out]
            n740 = local read "XY Graph 2"() -> (w1593:cluster{dbl[], dbl[]}[])
            n741 = local read "Slide 2"() -> (w1588:dbl)
            n742 = Decimate 1D Array(w1593) -> (w1590:cluster{dbl[], dbl[]}[], w1589:cluster{dbl[], dbl[]}[])
            n743 = local read "NumPts 2"() -> (w1594:dbl)
            n744 = Array To Cluster(array=w1590) -> (cluster=w1598:T8)
            n745 = Unbundle(w1598) -> ("[0]"=w1597:cluster{dbl[], dbl[]})  [unwired: 8 out]
            n746 = Unbundle(w1597) -> (w1596:dbl[], w1595:dbl[])
            n747 = Array Subset(array=w1596, index=w1588, length=w1594) -> (w1586:dbl[])
            n748 = Array Subset(array=w1595, index=w1588, length=w1594) -> (w1585:dbl[])
            n749 = local write "Index 2"(w1588) -> ()
            n750 = Bundle(w1586, w1585) -> (w1592:cluster{dbl[], dbl[]})  [unwired: 1 in]
            n751 = Build Array (concatenate)(w1590, w1589, w1592) -> (w1591:cluster{dbl[], dbl[]}[])
            n752 = local write "XY Graph 2"(w1591) -> ()
            n753 = local write "Array 7"(w1585) -> ()
            n754 = local write "Array 8"(w1586) -> ()
            n755 = call "sts_calc_subvi.vi"("Array 2"=w1586, "Array"=w1585) -> ("STS"=w1587:dbl)  [unwired: 9 in]
            n756 = local write "New: STS"(w1587) -> ()
          }
          event "Save Changes?": Mouse Down {
            n757 = event-data() -> ()  [unwired: 1 in, 5 out]
            n758 = flat-sequence {
              tunnel: [w1626] -> w1604
              tunnel: [w1625] -> w1602
              tunnel: [w1625] -> w1601
              tunnel: [w1608] -> w1599
              tunnel: w1604 -> [w1734]
              tunnel: [w1735] -> w1603
              tunnel: w1602 -> [w1735]
              tunnel: w1601 -> [w1733]
              tunnel: [w1731] -> w1600
              tunnel: w1599 -> [w1731]
              tunnel: w1603 -> [w1740]
              tunnel: w1600 -> [w1739]
              frame #0 {
                w1613 = -1
                w1606 = "S.T.S. (V/decade):"
                w1607 = "Threshold V (V):"
                (unwired) 3
                w1611 = 1
                n759 = local read "New: Mobility-Sat"() -> (w1648:dbl)
                n760 = local read "Data File"() -> (w1626:path)
                n761 = local read "New: Width"() -> (w1639:dbl)
                n762 = local read "New: Dielectric"() -> (w1649:dbl)
                n763 = local read "New: Length"() -> (w1637:dbl)
                n764 = flat-sequence {
                  tunnel: [w1662] -> w1605
                  tunnel: w1605 -> [w1679]
                  frame #0 {
                    # "Makes Empty File for Transformer Data"
                    n765 = local read "Data Folder"() -> (w1651:path)
                    n766 = Build Path(base path=w1651, name or relative path="Stats") -> (appended path=w1653:path)
                    n767 = call <vilib>:"Check if File or Folder Exists.vi"("path"=w1653) -> ("file or folder exists?"=w1654:bool, "dup path"=w1655:path)  [unwired: 8 in, 1 out]
                    n768 = case shown="False" w1654 {
                      tunnel: [w1659 w1661] -> w1656
                      tunnel: w1655 -> [w1660 w1661]
                      frame False {
                        n769 = Create Folder(path (use dialog)=w1660) -> (created path=w1659:path)  [unwired: 2 in, 2 out]
                      }
                      frame True {
                      }
                    }
                    n770 = Build Path(base path=w1656, name or relative path="Tranformer Data.txt") -> (appended path=w1658:path)
                    n771 = call-poly <vilib>:"Write To Spreadsheet File.vi"("append to file? (new file:F)"=TRUE, "file path (dialog if empty)"=w1658) -> ()  [unwired: 6 in, 1 out]
                  }
                  frame #1 {
                    # "Adds Headers if they don't exist"
                    n772 = Concatenate Strings("Stats\\", "Tranformer Data.txt") -> (w1669:string)
                    n773 = local read "Data Folder"() -> (w1668:path)
                    n774 = Build Path(base path=w1668, name or relative path=w1669) -> (appended path=w1662:path)
                    n775 = call-poly <vilib>:"Read From Spreadsheet File.vi"("file path (dialog if empty)"=w1662) -> ("first row"=w1667:string[])  [unwired: 6 in, 4 out]
                    n776 = Search 1D Array(1D array=w1667, element="DeviceID") -> (index of element=w1665:i32)  [unwired: 1 in]
                    n777 = Equal?(x=w1665, y=0) -> (x = y?=w1663:bool)
                    n778 = case shown="False" w1663 {
                      tunnel: w1662 -> [w1673 _]
                      frame False {
                        n779 = local read "Transformer \nHeaders"() -> (w1672:string[])
                        n780 = call-poly <vilib>:"Write To Spreadsheet File.vi"("1D data"=w1672, "file path (dialog if empty)"=w1673) -> ()  [unwired: 6 in, 1 out]
                      }
                      frame True {
                      }
                    }
                  }
                  frame #2 {
                    # "Adds current device if it doesn't exist"
                    n781 = local read "Current \nRecord"() -> (w1678:string[])
                    n782 = Index Array(array=w1678, index=0) -> (element=w1677:string)
                    n783 = Concatenate Strings("Stats\\", "Tranformer Data.txt") -> (w1682:string)
                    n784 = local read "Data Folder"() -> (w1681:path)
                    n785 = local write "Current Device ID"(w1677) -> ()
                    n786 = local read "Current Device ID"() -> (w1687:string)
                    n787 = Build Path(base path=w1681, name or relative path=w1682) -> (appended path=w1680:path)
                    n788 = call-poly <vilib>:"Read From Spreadsheet File.vi"("file path (dialog if empty)"=w1680) -> ("all rows"=w1674:string[][])  [unwired: 6 in, 4 out]
                    n789 = Index Array(array=w1674, index (col)=0) -> (element=w1675:string[])  [unwired: 1 in]
                    n790 = Search 1D Array(1D array=w1675, element=w1687) -> (index of element=w1676:i32)  [unwired: 1 in]
                    n791 = Equal?(x=w1676, y=-1) -> (x = y?=w1689:bool)
                    n792 = case shown="False" w1689 {
                      tunnel: w1679 -> [w1692 w1703]
                      tunnel: w1676 -> [w1695 _]
                      tunnel: w1674 -> [w1696 _]
                      frame False {
                        n793 = local read "Current \nRecord"() -> (w1694:string[])
                        n794 = Replace Array Subset(array=w1696, new element=w1694, index (row)=w1695) -> (w1693:string[][])  [unwired: 1 in]
                        n795 = flat-sequence {
                          tunnel: w1692 -> [w1697]
                          tunnel: w1693 -> [w1698]
                          tunnel: [w1698] -> w1691
                          tunnel: [w1697] -> w1690
                          tunnel: w1691 -> [w1700]
                          tunnel: w1690 -> [w1699]
                          frame #0 {
                            n796 = Delete(path (use dialog)=w1697) -> ()  [unwired: 4 in, 3 out]
                          }
                          frame #1 {
                            n797 = call-poly <vilib>:"Write To Spreadsheet File.vi"("append to file? (new file:F)"=TRUE, "2D data"=w1700, "file path (dialog if empty)"=w1699) -> ()  [unwired: 5 in, 1 out]
                          }
                        }
                      }
                      frame True {
                        n798 = local read "Current \nRecord"() -> (w1702:string[])
                        n799 = call-poly <vilib>:"Write To Spreadsheet File.vi"("append to file? (new file:F)"=TRUE, "1D data"=w1702, "file path (dialog if empty)"=w1703) -> ()  [unwired: 5 in, 1 out]
                      }
                    }
                  }
                }
                n800 = call-poly <vilib>:"Read From Spreadsheet File.vi"("file path (dialog if empty)"=w1626) -> ("all rows"=w1618:string[][])  [unwired: 6 in, 4 out]
                n801 = Number To Fractional String(number=w1637) -> (F-format string=w1629:string)  [unwired: 3 in]
                n802 = Replace Array Subset(array=w1618, new element=w1629, index (row)=12, index (col)=w1611) -> (w1633:string[][])
                n803 = Number To Fractional String(number=w1639) -> (F-format string=w1640:string)  [unwired: 3 in]
                n804 = Replace Array Subset(array=w1633, new element=w1640, index (row)=13, index (col)=w1611) -> (w1635:string[][])
                n805 = Number To Fractional String(number=w1648) -> (F-format string=w1627:string)  [unwired: 3 in]
                n806 = Number To Fractional String(number=w1649) -> (F-format string=w1628:string)  [unwired: 3 in]
                n807 = Number To Decimal String(number=w1637) -> (decimal integer string=w1636:string)  [unwired: 1 in]
                n808 = Strip Path(path=w1626) -> (stripped path=w1647:path)  [unwired: 1 out]
                n809 = local read "Index"() -> (w1642:string)
                n810 = Replace Array Subset(array=w1635, new element=w1627, index (row)=15, index (col)=w1611) -> (w1634:string[][])
                n811 = Number To Decimal String(number=w1639) -> (decimal integer string=w1638:string)  [unwired: 1 in]
                n812 = Path To String(path=w1647) -> (string=w1645:string)
                n813 = Replace Array Subset(array=w1634, new element=w1628, index (row)=7, index (col)=w1611) -> (w1610:string[][])
                n814 = call "Build Text"("Index"=w1642, "Length"=w1636, "Width"=w1638) -> ("Result"=w1643:string)  [unwired: 11 in, 1 out]
                n815 = Concatenate Strings(w1645, "\\", w1643) -> (w1644:string)
                n816 = String To Path(string=w1644) -> (path=w1625:path)
                n817 = Array Size(array=w1618) -> (size(s)=w1620:i32[])
                n818 = Index Array(array=w1620, index=0) -> (element=w1619:i32)
                n819 = Array Subset(array=w1618, index (row)=0, index (col)=0) -> (w1624:string[][])  [unwired: 2 in]
                n820 = Reshape Array(w1624, w1619) -> (w1612:string[])
                n821 = Search 1D Array(1D array=w1612, element=w1607) -> (index of element=w1616:i32)  [unwired: 1 in]
                n822 = Search 1D Array(1D array=w1612, element=w1606) -> (index of element=w1617:i32)  [unwired: 1 in]
                n823 = Equal?(x=w1616, y=w1613) -> (x = y?=w1614:bool)
                n824 = Equal?(x=w1617, y=w1613) -> (x = y?=w1615:bool)
                n825 = case shown="True" w1614 {
                  tunnel: w1616 -> [_ _]
                  tunnel: w1610 -> [w1721 w1729]
                  tunnel: [w1720 w1728] -> w1609
                  tunnel: w1607 -> [_ w1727]
                  frame False {
                    n826 = local read "New: VT"() -> (w1723:dbl)
                    n827 = Number To Fractional String(number=w1723) -> (F-format string=w1719:string)  [unwired: 3 in]
                    n828 = Replace Array Subset(array=w1721, new element=w1719, index (row)=17, index (col)=1) -> (w1720:string[][])
                  }
                  frame True {
                    n829 = local read "New: VT"() -> (w1730:dbl)
                    n830 = Number To Fractional String(number=w1730) -> (F-format string=w1726:string)  [unwired: 3 in]
                    n831 = Build Array(w1727, w1726) -> (w1725:string[])
                    n832 = Insert Into Array(array=w1729, index (row)=17, new element=w1725) -> (w1728:string[][])  [unwired: 1 in]
                  }
                }
                n833 = case shown="True" w1615 {
                  tunnel: w1617 -> [_ _]
                  tunnel: w1609 -> [w1708 w1716]
                  tunnel: [w1707 w1715] -> w1608
                  tunnel: w1606 -> [_ w1713]
                  frame False {
                    n834 = local read "New: STS"() -> (w1710:dbl)
                    n835 = Number To Fractional String(number=w1710) -> (F-format string=w1706:string)  [unwired: 3 in]
                    n836 = Replace Array Subset(array=w1708, new element=w1706, index (row)=18, index (col)=1) -> (w1707:string[][])
                  }
                  frame True {
                    n837 = local read "New: STS"() -> (w1717:dbl)
                    n838 = Number To Fractional String(number=w1717) -> (F-format string=w1714:string)  [unwired: 3 in]
                    n839 = Build Array(w1713, w1714) -> (w1712:string[])
                    n840 = Insert Into Array(array=w1716, index (row)=18, new element=w1712) -> (w1715:string[][])  [unwired: 1 in]
                  }
                }
              }
              frame #1 {
                n841 = Equal?(x=w1734, y=w1733) -> (x = y?=w1732:bool)
                n842 = case shown="False" w1732 {
                  tunnel: w1734 -> [w1738 _]
                  tunnel: w1733 -> [w1737 _]
                  frame False {
                    n843 = Move(source path=w1738, 9:TRUE, 10:w1737) -> ()  [unwired: 2 in, 3 out]
                  }
                  frame True {
                  }
                }
              }
              frame #2 {
                n844 = local write "Data File"(w1740) -> ()
                n845 = call-poly <vilib>:"Write To Spreadsheet File.vi"("2D data"=w1739, "file path (dialog if empty)"=w1740) -> ()  [unwired: 6 in, 1 out]
              }
            }
          }
          event "Save Changes? 2": Mouse Down {
            n846 = event-data() -> ()  [unwired: 1 in, 5 out]
            n847 = stacked-sequence {
              seq-local: [w1817 _ _ _ _] -> [_ w1870 _ _ _]
              seq-local: [w1816 _ _ _ _] -> [_ w1871 _ _ _]
              seq-local: [w1816 _ _ _ _] -> [_ w1869 _ _ _]
              seq-local: [w1799 _ _ _ _] -> [_ w1867 _ _ _]
              seq-local: [_ w1871 _ _ _] -> [_ _ w1876 _ _]
              seq-local: [_ w1867 _ _ _] -> [_ _ w1875 _ _]
              frame #0 {
                w1804 = -1
                w1797 = "S.T.S. (V/decade):"
                w1798 = "Threshold V (V):"
                (unwired) 3
                w1802 = 1
                n848 = local read "Data File"() -> (w1817:path)
                n849 = local read "New: Width"() -> (w1830:dbl)
                n850 = local read "New: Dielectric"() -> (w1840:dbl)
                n851 = local read "New: Length"() -> (w1828:dbl)
                n852 = local read "New: Mobility-Sat"() -> (w1839:dbl)
                n853 = call-poly <vilib>:"Read From Spreadsheet File.vi"("file path (dialog if empty)"=w1817) -> ("all rows"=w1809:string[][])  [unwired: 6 in, 4 out]
                n854 = Number To Fractional String(number=w1828) -> (F-format string=w1820:string)  [unwired: 3 in]
                n855 = Replace Array Subset(array=w1809, new element=w1820, index (row)=12, index (col)=w1802) -> (w1824:string[][])
                n856 = Number To Fractional String(number=w1830) -> (F-format string=w1831:string)  [unwired: 3 in]
                n857 = Replace Array Subset(array=w1824, new element=w1831, index (row)=13, index (col)=w1802) -> (w1826:string[][])
                n858 = Number To Fractional String(number=w1839) -> (F-format string=w1818:string)  [unwired: 3 in]
                n859 = Number To Fractional String(number=w1840) -> (F-format string=w1819:string)  [unwired: 3 in]
                n860 = Number To Decimal String(number=w1828) -> (decimal integer string=w1827:string)  [unwired: 1 in]
                n861 = Strip Path(path=w1817) -> (stripped path=w1838:path)  [unwired: 1 out]
                n862 = local read "Index"() -> (w1833:string)
                n863 = Replace Array Subset(array=w1826, new element=w1818, index (row)=15, index (col)=w1802) -> (w1825:string[][])
                n864 = Number To Decimal String(number=w1830) -> (decimal integer string=w1829:string)  [unwired: 1 in]
                n865 = Path To String(path=w1838) -> (string=w1836:string)
                n866 = Replace Array Subset(array=w1825, new element=w1819, index (row)=7, index (col)=w1802) -> (w1801:string[][])
                n867 = call "Build Text2"("Index"=w1833, "Length"=w1827, "Width"=w1829) -> ("Result"=w1834:string)  [unwired: 11 in, 1 out]
                n868 = Concatenate Strings(w1836, "\\", w1834) -> (w1835:string)
                n869 = String To Path(string=w1835) -> (path=w1816:path)
                n870 = Array Size(array=w1809) -> (size(s)=w1811:i32[])
                n871 = Index Array(array=w1811, index=0) -> (element=w1810:i32)
                n872 = Array Subset(array=w1809, index (row)=0, index (col)=0) -> (w1815:string[][])  [unwired: 2 in]
                n873 = Reshape Array(w1815, w1810) -> (w1803:string[])
                n874 = Search 1D Array(1D array=w1803, element=w1798) -> (index of element=w1807:i32)  [unwired: 1 in]
                n875 = Search 1D Array(1D array=w1803, element=w1797) -> (index of element=w1808:i32)  [unwired: 1 in]
                n876 = Equal?(x=w1807, y=w1804) -> (x = y?=w1805:bool)
                n877 = Equal?(x=w1808, y=w1804) -> (x = y?=w1806:bool)
                n878 = case shown="True" w1805 {
                  tunnel: w1807 -> [_ _]
                  tunnel: w1801 -> [w1857 w1865]
                  tunnel: [w1856 w1864] -> w1800
                  tunnel: w1798 -> [_ w1863]
                  frame False {
                    n879 = local read "New: VT"() -> (w1859:dbl)
                    n880 = Number To Fractional String(number=w1859) -> (F-format string=w1855:string)  [unwired: 3 in]
                    n881 = Replace Array Subset(array=w1857, new element=w1855, index (row)=17, index (col)=1) -> (w1856:string[][])
                  }
                  frame True {
                    n882 = local read "New: VT"() -> (w1866:dbl)
                    n883 = Number To Fractional String(number=w1866) -> (F-format string=w1862:string)  [unwired: 3 in]
                    n884 = Build Array(w1863, w1862) -> (w1861:string[])
                    n885 = Insert Into Array(array=w1865, index (row)=17, new element=w1861) -> (w1864:string[][])  [unwired: 1 in]
                  }
                }
                n886 = case shown="True" w1806 {
                  tunnel: w1808 -> [_ _]
                  tunnel: w1800 -> [w1844 w1852]
                  tunnel: [w1843 w1851] -> w1799
                  tunnel: w1797 -> [_ w1849]
                  frame False {
                    n887 = local read "New: STS"() -> (w1846:dbl)
                    n888 = Number To Fractional String(number=w1846) -> (F-format string=w1842:string)  [unwired: 3 in]
                    n889 = Replace Array Subset(array=w1844, new element=w1842, index (row)=18, index (col)=1) -> (w1843:string[][])
                  }
                  frame True {
                    n890 = local read "New: STS"() -> (w1853:dbl)
                    n891 = Number To Fractional String(number=w1853) -> (F-format string=w1850:string)  [unwired: 3 in]
                    n892 = Build Array(w1849, w1850) -> (w1848:string[])
                    n893 = Insert Into Array(array=w1852, index (row)=18, new element=w1848) -> (w1851:string[][])  [unwired: 1 in]
                  }
                }
              }
              frame #1 {
                n894 = Equal?(x=w1870, y=w1869) -> (x = y?=w1868:bool)
                n895 = case shown="False" w1868 {
                  tunnel: w1870 -> [w1874 _]
                  tunnel: w1869 -> [w1873 _]
                  frame False {
                    n896 = Move(source path=w1874, 9:TRUE, 10:w1873) -> ()  [unwired: 2 in, 3 out]
                  }
                  frame True {
                  }
                }
              }
              frame #2 {
                n897 = local write "Data File"(w1876) -> ()
                n898 = call-poly <vilib>:"Write To Spreadsheet File.vi"("2D data"=w1875, "file path (dialog if empty)"=w1876) -> ()  [unwired: 6 in, 1 out]
              }
              frame #3 {
                w1941 = 0
                # "Moves to next file and displays new image/data"
                n899 = local read "NumPts 2"() -> (w1900:dbl)
                n900 = local read "Folder Index"() -> (w1878:dbl)
                n901 = local read "NumPts"() -> (w1907:dbl)
                n902 = local read "Row Start"() -> (w1906:dbl)
                n903 = local read "Data File"() -> (w1946:path)
                n904 = property on="Image Out" class="ImageControl"() -> (error out=w1882:errorcluster, "Image Center Position"=w1886:cluster{"X":u32, "Y":u32})  [unwired: 2 in, 1 out]
                n905 = Strip Path(path=w1946) -> (stripped path=w1937:path, name=w1958:string)
                n906 = local write "Data Folder"(w1937) -> ()
                n907 = List Folder(path=w1937) -> (filenames=w1951:string[])  [unwired: 3 in, 3 out]
                n908 = Unbundle(w1886) -> ("X"=w1884:u32)  [unwired: 1 out]
                n909 = Array Size(array=w1951) -> (size(s)=w1947:i32)
                n910 = Path To String(path=w1937) -> (string=w1959:string)
                n911 = Search 1D Array(1D array=w1951, element=w1958) -> (index of element=w1948:i32)  [unwired: 1 in]
                n912 = Bundle("X"=w1884, 0) -> (w1885:cluster{"X":u32, i32})  [unwired: 1 in]
                n913 = Unbundle() -> ("Vt"=w1893, "STS"=w1892, "On/Off"=w1891)  [unwired: 1 in]
                n914 = local write "Rec: On/Off"(w1891) -> ()
                n915 = Decrement(x=w1947) -> (x-1=w1949:i32)
                n916 = Equal?(x=w1948, y=w1949) -> (x = y?=w1950:bool)
                n917 = case shown="False" w1950 {
                  tunnel: w1878 -> [w2081 _]
                  tunnel: [w2080 0] -> w1877
                  frame False {
                    n918 = Increment(x=w2081) -> (x+1=w2080:dbl)
                  }
                  frame True {
                  }
                }
                n919 = Index Array(array=w1951, index=w1877) -> (element=w1952:string)
                n920 = local write "Data Name"(w1952) -> ()
                n921 = Concatenate Strings(w1959, "\\", w1952) -> (w1957:string)
                n922 = property on="Image Out" class="ImageControl"(error in=w1882, "Image Center Position"=w1885) -> ()  [unwired: 1 in, 2 out]
                n923 = String To Path(string=w1957) -> (path=w1908:path)
                n924 = call "sub_thresh_swing_subvi.vi"("Path"=w1908, "NumPts"=w1900, "Row Start"=w1906) -> ("Index"=w1901:dbl, "XY Graph"=w1896:cluster{dbl[], dbl[]}[], "Sub Threshold Swing"=w1909:dbl)  [unwired: 8 in, 2 out]
                n925 = Decimate 1D Array(w1896) -> (w1899:cluster{dbl[], dbl[]}[])  [unwired: 1 out]
                n926 = Array To Cluster(array=w1899) -> (cluster=w1897:T8)
                n927 = Unbundle(w1897) -> ("[0]"=w1898:cluster{dbl[], dbl[]})  [unwired: 8 out]
                n928 = Unbundle(w1898) -> (w1895:dbl[], w1894:dbl[])
                n929 = local write "Calc: STS"(w1909) -> ()
                n930 = local write "XY Graph 2"(w1896) -> ()
                n931 = local write "Index 2"(w1901) -> ()
                n932 = call "mobility_subvi_07_12a_JW.vi"("Path"=w1908, "NumPts"=w1907, 11:w1906) -> ("Dielectric (d)"=w1912:dbl, "Index"=w1917:dbl, "XY Graph"=w1920:cluster{dbl[], dbl[]}[], "Length"=w1910:dbl, "Vt"=w1913:dbl, "Width"=w1911:dbl, "Table Control"=w1955:string[][], "Table Control 2"=w1954:string[][], "Mobility"=w1953:dbl)  [unwired: 3 in, 1 out]
                n933 = local write "Rec: Dielectric (d)"(w1912) -> ()
                n934 = local write "Calc: VT"(w1913) -> ()
                n935 = local write "New: Dielectric"(w1912) -> ()
                n936 = Decimate 1D Array(w1920) -> (w1921:cluster{dbl[], dbl[]}[])  [unwired: 1 out]
                n937 = Array To Cluster(array=w1921) -> (cluster=w1923:T8)
                n938 = local write "Table Control"(w1955) -> ()
                n939 = Unbundle(w1923) -> ("[0]"=w1922:cluster{dbl[], dbl[]})  [unwired: 8 out]
                n940 = Unbundle(w1922) -> (w1903:dbl[], w1902:dbl[])
                n941 = local write "Calc: Mobility-Sat"(w1953) -> ()
                n942 = local write "XY Graph"(w1920) -> ()
                n943 = local write "Table Control 2"(w1954) -> ()
                n944 = Array Subset(array=w1903, index=w1917, length=w1907) -> (w1919:dbl[])
                n945 = Array Subset(array=w1902, index=w1917, length=w1907) -> (w1918:dbl[])
                n946 = local write "Rec: Width"(w1911) -> ()
                n947 = local write "Rec: Length"(w1910) -> ()
                n948 = local write "Array 2"(w1918) -> ()
                n949 = local write "Array"(w1919) -> ()
                n950 = local write "Device Index"(w1917) -> ()
                n951 = local write "Slide"(w1917) -> ()
                n952 = local write "Rec: STS"(w1892) -> ()
                n953 = local write "Rec: VT"(w1893) -> ()
                n954 = Array Subset(array=w1895, index=w1901, length=w1900) -> (w1905:dbl[])
                n955 = Array Subset(array=w1894, index=w1901, length=w1900) -> (w1904:dbl[])
                n956 = local write "New: Width"(w1911) -> ()
                n957 = local write "Data File"(w1908) -> ()
                n958 = local write "New: Length"(w1910) -> ()
                n959 = local write "Folder Index"(w1877) -> ()
                n960 = local write "Array 8"(w1905) -> ()
                n961 = local write "Array 7"(w1904) -> ()
                n962 = call-poly <vilib>:"Read From Spreadsheet File.vi"("file path (dialog if empty)"=w1908) -> ("all rows"=w1943:string[][])  [unwired: 6 in, 4 out]
                n963 = local read "Image Folder"() -> (w1931:path)
                n964 = Array Size(array=w1943) -> (size(s)=w1942:i32[])
                n965 = List Folder(path=w1931) -> (filenames=w1936:string[])  [unwired: 3 in, 3 out]
                n966 = Index Array(array=w1942, index=w1941) -> (element=w1915:i32)
                n967 = Subtract(x=w1915, y=20) -> (x-y=w1914:i32)
                n968 = property on="Slide" class="Slide (strict)"("Scale.Maximum"=w1914) -> ()  [unwired: 2 in, 2 out]
                n969 = Array Subset(array=w1943, index (row)=w1941, index (col)=w1941, length (col)=3) -> (w1944:string[][])  [unwired: 1 in]
                n970 = Reshape Array(w1944, w1915) -> (w1924:string[])
                n971 = Search 1D Array(1D array=w1924, element="Mobility-Sat (cm^2/Vs):") -> (index of element=w1929:i32)  [unwired: 1 in]
                n972 = Search 1D Array(1D array=w1924, element="Index:") -> (index of element=w1938:i32)  [unwired: 1 in]
                n973 = Increment(x=w1938) -> (x+1=w1939:i32)
                n974 = Index Array(array=w1924, index=w1939) -> (element=w1934:string)
                n975 = while {
                  tunnel: w1936 -> [w1967]
                  tunnel: w1934 -> [w1965]
                  tunnel: [w1964] -> _
                  tunnel: [w1964] -> w1935
                  tunnel: w1915 -> [w1963]
                  i -> [w1964]
                  stop <- w1960 stop-if-true
                  n976 = Index Array(array=w1967, index=w1964) -> (element=w1968:string)
                  n977 = xnode "Match Regular Expression"("input string"=w1968, "regular expression"=w1965) -> ("whole match"=w1966:string)  [unwired: 4 in, 4 out]
                  n978 = Equal?(x=w1966, y=w1965) -> (x = y?=w1962:bool)
                  n979 = Equal?(x=w1963, y=w1964) -> (x = y?=w1961:bool)
                  n980 = Or(x=w1962, y=w1961) -> (x .or. y?=w1960:bool)
                }
                n981 = local write "Index"(w1934) -> ()
                n982 = Increment(x=w1929) -> (x+1=w1928:i32)
                n983 = local read "No Image"() -> (w1887:path)
                n984 = Index Array(array=w1924, index=w1928) -> (element=w1926:string)
                n985 = Fract/Exp String To Number(string=w1926) -> (number=w1925:dbl)  [unwired: 3 in, 1 out]
                n986 = local write "Rec: Mobility-Sat"(w1925) -> ()
                n987 = Path To String(path=w1931) -> (string=w1933:string)
                n988 = local read "Image Out"() -> (w1879:T2)
                n989 = Index Array(array=w1936, index=w1935) -> (element=w1889:string)
                n990 = Empty String/Path?(string/path=w1889) -> (empty?=w1890:bool)
                n991 = Concatenate Strings(w1933, "\\", w1889) -> (w1932:string)
                n992 = local write "Image Name"(w1889) -> ()
                n993 = String To Path(string=w1932) -> (path=w1888:path)
                n994 = Select(t=w1887, s=w1890, f=w1888) -> (s? t:f=w1881:path)
                n995 = local write "Image File"(w1881) -> ()
                n996 = call "IMAQ ReadFile"("File Path"=w1881, "Image"=w1879) -> ("Image Out"=w1880:T2)  [unwired: 5 in, 4 out]
                n997 = local write "Image Out 2"(w1880) -> ()
                n998 = local write "Image Out"(w1880) -> ()
                n999 = invoke on="Image Out" class="ImageControl" method="Clear ROI"() -> ()  [unwired: 3 in, 3 out]
              }
              frame #4 {
                # "Output ROI data"
                n1000 = local read "Image Folder"() -> (w2083:path)
                n1001 = Build Path(base path=w2083, name or relative path="ROI") -> (appended path=w2085:path)
                n1002 = local read "Index"() -> (w2084:string)
                n1003 = Build Path(base path=w2085, name or relative path=w2084) -> (appended path=w2090:path)
                n1004 = invoke on="Image Out" class="ImageControl" method="Clear ROI"() -> (error out=w2089:errorcluster)  [unwired: 3 in, 2 out]
                n1005 = call <vilib>:"Check if File or Folder Exists.vi"("error in (no error)"=w2089, "path"=w2090) -> ("file or folder exists?"=w2087:bool, "dup path"=w2088:path)  [unwired: 7 in, 1 out]
                n1006 = case shown="True" w2087 {
                  tunnel: w2088 -> [_ w2091]
                  frame False {
                  }
                  frame True {
                    n1007 = Read from Text File(file (use dialog)=w2091) -> (text=w2095:string)  [unwired: 3 in, 3 out]
                    n1008 = property on="Image Out" class="ImageControl"() -> ("ROI"=w2092:T9)  [unwired: 2 in, 2 out]
                    n1009 = Unflatten From String(type=w2092, binary string=w2095) -> (value=w2093:T9, error out=w2094:errorcluster)  [unwired: 3 in, 1 out]
                    n1010 = property on="Image Out" class="ImageControl"(error in=w2094, "ROI"=w2093) -> ()  [unwired: 1 in, 2 out]
                  }
                }
              }
            }
            n1011 = flat-sequence {
              tunnel: [w1754] -> w1741
              tunnel: w1741 -> [w1768]
              frame #0 {
                # "Makes Empty File for Transformer Data"
                n1012 = local read "Data Folder"() -> (w1743:path)
                n1013 = Build Path(base path=w1743, name or relative path="Stats") -> (appended path=w1745:path)
                n1014 = call <vilib>:"Check if File or Folder Exists.vi"("path"=w1745) -> ("file or folder exists?"=w1746:bool, "dup path"=w1747:path)  [unwired: 8 in, 1 out]
                n1015 = case shown="False" w1746 {
                  tunnel: [w1751 w1753] -> w1748
                  tunnel: w1747 -> [w1752 w1753]
                  frame False {
                    n1016 = Create Folder(path (use dialog)=w1752) -> (created path=w1751:path)  [unwired: 2 in, 2 out]
                  }
                  frame True {
                  }
                }
                n1017 = Build Path(base path=w1748, name or relative path="Tranformer Data.txt") -> (appended path=w1750:path)
                n1018 = call-poly <vilib>:"Write To Spreadsheet File.vi"("append to file? (new file:F)"=TRUE, "file path (dialog if empty)"=w1750) -> ()  [unwired: 6 in, 1 out]
              }
              frame #1 {
                # "Adds Headers if they don't exist"
                n1019 = Concatenate Strings("Stats\\", "Tranformer Data.txt") -> (w1761:string)
                n1020 = local read "Data Folder"() -> (w1760:path)
                n1021 = Build Path(base path=w1760, name or relative path=w1761) -> (appended path=w1754:path)
                n1022 = call-poly <vilib>:"Read From Spreadsheet File.vi"("file path (dialog if empty)"=w1754) -> ("first row"=w1759:string[])  [unwired: 6 in, 4 out]
                n1023 = Search 1D Array(1D array=w1759, element="DeviceID") -> (index of element=w1757:i32)  [unwired: 1 in]
                n1024 = Equal?(x=w1757, y=0) -> (x = y?=w1755:bool)
                n1025 = case shown="False" w1755 {
                  tunnel: w1754 -> [w1765 _]
                  frame False {
                    n1026 = local read "Transformer \nHeaders"() -> (w1764:string[])
                    n1027 = call-poly <vilib>:"Write To Spreadsheet File.vi"("1D data"=w1764, "file path (dialog if empty)"=w1765) -> ()  [unwired: 6 in, 1 out]
                  }
                  frame True {
                  }
                }
              }
              frame #2 {
                # "Adds current device if it doesn't exist"
                n1028 = local read "Current \nRecord"() -> (w1771:string[])
                n1029 = Index Array(array=w1771, index=0) -> (element=w1770:string)
                n1030 = Concatenate Strings("Stats\\", "Tranformer Data.txt") -> (w1774:string)
                n1031 = local read "Data Folder"() -> (w1773:path)
                n1032 = local write "Current Device ID"(w1770) -> ()
                n1033 = local read "Current Device ID"() -> (w1780:string)
                n1034 = Build Path(base path=w1773, name or relative path=w1774) -> (appended path=w1772:path)
                n1035 = call-poly <vilib>:"Read From Spreadsheet File.vi"("file path (dialog if empty)"=w1772) -> ("all rows"=w1767:string[][])  [unwired: 6 in, 4 out]
                n1036 = Index Array(array=w1767, index (col)=0) -> (element=w1778:string[])  [unwired: 1 in]
                n1037 = Search 1D Array(1D array=w1778, element=w1780) -> (index of element=w1766:i32)  [unwired: 1 in]
                n1038 = Equal?(x=w1766, y=-1) -> (x = y?=w1769:bool)
                n1039 = case shown="False" w1769 {
                  tunnel: w1768 -> [w1782 w1795]
                  tunnel: w1766 -> [w1787 _]
                  tunnel: w1767 -> [w1788 _]
                  frame False {
                    n1040 = local read "Current \nRecord"() -> (w1786:string[])
                    n1041 = Replace Array Subset(array=w1788, new element=w1786, index (row)=w1787) -> (w1783:string[][])  [unwired: 1 in]
                    n1042 = flat-sequence {
                      tunnel: [w1789] -> _
                      tunnel: [w1790] -> _
                      tunnel: [w1790] -> w1785
                      tunnel: [w1789] -> w1784
                      tunnel: w1783 -> [w1790]
                      tunnel: w1782 -> [w1789]
                      tunnel: w1785 -> [w1792]
                      tunnel: w1784 -> [w1791]
                      frame #0 {
                        n1043 = Delete(path (use dialog)=w1789) -> ()  [unwired: 4 in, 3 out]
                      }
                      frame #1 {
                        n1044 = call-poly <vilib>:"Write To Spreadsheet File.vi"("append to file? (new file:F)"=TRUE, "2D data"=w1792, "file path (dialog if empty)"=w1791) -> ()  [unwired: 5 in, 1 out]
                      }
                    }
                  }
                  frame True {
                    n1045 = local read "Current \nRecord"() -> (w1794:string[])
                    n1046 = call-poly <vilib>:"Write To Spreadsheet File.vi"("append to file? (new file:F)"=TRUE, "1D data"=w1794, "file path (dialog if empty)"=w1795) -> ()  [unwired: 5 in, 1 out]
                  }
                }
              }
            }
          }
          event "Export": Mouse Down {
            n1047 = event-data() -> ()  [unwired: 1 in, 7 out]
            n1048 = call "OA_ConnectToOrigin.vi"() -> ("error out"=w2117:errorcluster, "Origin.IOApplication"=w2118:refnum<k7>)  [unwired: 8 in]
            n1049 = local read "Data Folder"() -> (w2096:path)
            n1050 = local read "Project"() -> (w2116:path)
            n1051 = call "OA_Load.vi"("error in (no error)"=w2117, "Path"=w2116, "Origin.IOApplication"=w2118) -> ("error out"=w2109:errorcluster, "Origin.IOApplication"=w2110:refnum<k7>)  [unwired: 1 out]
            n1052 = call "OAExecute.vi"("script"="document -m 3;", "Error IO"=w2109, "Origin.IOApplication"=w2110) -> ("Error IO Out"=w2107:errorcluster, "Origin.IOApplication"=w2108:refnum<k7>)  [unwired: 1 in, 1 out]
            n1053 = Build Path(base path=w2096, name or relative path="Stats") -> (appended path=w2097:path)
            n1054 = flat-sequence {
              tunnel: w2096 -> [w2138]
              tunnel: w2115 -> [w2137]
              tunnel: [w2127] -> w2120
              tunnel: [w2128] -> w2119
              tunnel: w2108 -> [w2132]
              tunnel: w2107 -> [w2131]
              tunnel: w2096 -> [w2154]
              tunnel: w2115 -> [w2153]
              tunnel: w2120 -> [w2149]
              tunnel: w2119 -> [w2150]
              tunnel: [w2144] -> w2114
              tunnel: [w2143] -> w2113
              tunnel: w2096 -> [w2165]
              tunnel: w2115 -> [w2164]
              tunnel: w2114 -> [w2160]
              tunnel: w2113 -> [w2159]
              tunnel: [w2158] -> w2112
              tunnel: [w2157] -> w2111
              tunnel: w2096 -> [w2180]
              tunnel: w2115 -> [w2179]
              tunnel: w2112 -> [w2174]
              tunnel: w2111 -> [w2173]
              tunnel: [w2171] -> w2105
              tunnel: [w2170] -> w2104
              frame #0 {
                n1055 = call "Param_Analysis.vi"("error in (no error)"=w2131, "Folder 2"=w2138, "Parameter String"="Mobility (cm^2/Vs):", "Parameter Name"="Mobility", "Folder"=w2137) -> ("error out"=w2134:errorcluster, "Array 4"=w2124:string[], "Array 3"=w2133:string[][])  [unwired: 3 in, 1 out]
                n1056 = call "Origin_Export.vi"("String 3"="[MobHistTab]Sheet1", "error in (no error)"=w2134, "Array"=w2133, "String 2"="[MOBvsLTable]Mobilities", "String"="pe_cd \"Mobility Chart\";", "Origin.IOApplication"=w2132, "Array 2"=w2124) -> ("reference out"=w2130:refnum<k7>, "error out"=w2129:errorcluster)  [unwired: 2 in, 1 out]
                n1057 = call "OAExecute.vi"("script"="window -a MOBvsLTable;\nwindow -s TV;", "Error IO"=w2129, "Origin.IOApplication"=w2130) -> ("Error IO Out"=w2127:errorcluster, "Origin.IOApplication"=w2128:refnum<k7>)  [unwired: 1 in, 1 out]
              }
              frame #1 {
                n1058 = call "Param_Analysis.vi"("error in (no error)"=w2149, "Folder 2"=w2154, "Parameter String"="On/Off Current:", "Parameter Name"="On_Off_Current", "Folder"=w2153) -> ("error out"=w2148:errorcluster, "Array 4"=w2142:string[], "Array 3"=w2145:string[][])  [unwired: 3 in, 1 out]
                n1059 = call "Origin_Export.vi"("String 3"="[OnOffHistTab]Sheet1", "error in (no error)"=w2148, "Array"=w2145, "String 2"="[OnOffTable]On/Off Ratios", "String"="pe_cd \"OnOff vs L\";", "Origin.IOApplication"=w2150, "Array 2"=w2142) -> ("reference out"=w2144:refnum<k7>, "error out"=w2143:errorcluster)  [unwired: 2 in, 1 out]
              }
              frame #2 {
                n1060 = call "Param_Analysis.vi"("Folder 2"=w2165, "Parameter String"="S.T.S. (V/decade):", "Parameter Name"="STS", "Folder"=w2164) -> ("Array 4"=w2156:string[], "Array 3"=w2161:string[][])  [unwired: 4 in, 2 out]
                n1061 = call "Origin_Export.vi"("String 3"="[SHistTab]Sheet1", "error in (no error)"=w2159, "Array"=w2161, "String 2"="[STable]Threshold Swing", "String"="pe_cd \"Threshold Swing vs L\";", "Origin.IOApplication"=w2160, "Array 2"=w2156) -> ("reference out"=w2157:refnum<k7>, "error out"=w2158:errorcluster)  [unwired: 2 in, 1 out]
              }
              frame #3 {
                n1062 = call "Param_Analysis.vi"("Folder 2"=w2180, "Parameter String"="Threshold V (V):", "Parameter Name"="Threshold_V", "Folder"=w2179) -> ("Array 4"=w2169:string[], "Array 3"=w2172:string[][])  [unwired: 4 in, 2 out]
                n1063 = call "Origin_Export.vi"("String 3"="[VtHistTab]Sheet1", "error in (no error)"=w2174, "Array"=w2172, "String 2"="[VtTable]Threshold Voltages", "String"="pe_cd \"Threshold Voltage vs L\";", "Origin.IOApplication"=w2173, "Array 2"=w2169) -> ("reference out"=w2171:refnum<k7>, "error out"=w2170:errorcluster)  [unwired: 2 in, 1 out]
              }
            }
            n1064 = call <vilib>:"Check if File or Folder Exists.vi"("path"=w2097) -> ("file or folder exists?"=w2122:bool, "dup path"=w2121:path)  [unwired: 8 in, 1 out]
            n1065 = case shown="False" w2122 {
              tunnel: w2121 -> [w2182 w2183]
              tunnel: [w2181 w2183] -> w2115
              frame False {
                n1066 = Create Folder(path (use dialog)=w2182) -> (created path=w2181:path)  [unwired: 2 in, 2 out]
              }
              frame True {
              }
            }
            n1067 = call "File Dialog"("start path"=w2097) -> ("selected path"=w2100:path)  [unwired: 11 in, 3 out]
            n1068 = Path To String(path=w2100) -> (string=w2099:string)
            n1069 = call "OAExecute.vi"("script"="pe_cd /;\npe_cd \"Mobility Chart\"; ", "Error IO"=w2104, "Origin.IOApplication"=w2105) -> ("Error IO Out"=w2101:errorcluster, "Origin.IOApplication"=w2102:refnum<k7>)  [unwired: 1 in, 1 out]
            n1070 = call "OASaveProject.vi"("path"=w2099, "Error IO"=w2101, "Origin.IOApplication"=w2102) -> ()  [unwired: 3 out]
          }
          event "Blank Button": Mouse Down {
            n1071 = event-data() -> ()  [unwired: 1 in, 7 out]
            n1072 = local read "Data File"() -> (w2191:path)
            n1073 = Strip Path(path=w2191) -> (stripped path=w2187:path, name=w2189:string)
            n1074 = Path To String(path=w2187) -> (string=w2186:string)
            n1075 = Concatenate Strings(w2186, "\\", "X_", w2189) -> (w2185:string)
            n1076 = String To Path(string=w2185) -> (path=w2184:path)
            n1077 = Move(source path=w2191, 10:w2184) -> ()  [unwired: 3 in, 3 out]
            n1078 = local write "Data File"(w2184) -> ()
          }
          event "Cancel Button": Mouse Down {
            (unwired) 6
            n1079 = event-data() -> ()  [unwired: 1 in, 7 out]
            n1080 = call "Simulate_Keyboard.vi"("Action"=2, "Virtual Key"=162) -> ()  [unwired: 7 in, 1 out]
          }
        }
        n1081 = Reciprocal(x=w496) -> (1/x=w495:sgl)
        n1082 = Multiply(x=w495, y=10) -> (x*y=w497:sgl)
        n1083 = case shown="\"EQUALS\"" w536 {
          tunnel: w510 -> [w585 w591 w595 w597 w601 w603 w605 w607 w609 w611 w613 w615 w617 w619 w621 w623 w625 w627 w629 w631 w633 w635 w637 w639 w641 w643 w645 w647 w649 w651 w653 w655 w657 w659 w661 w663 w665 w667 w669 w671 w673 w675 w677 w679 w681 w683 w685 w687 w689 w691 w693 w695 w697 w699 w701 w703 w705 w707 w709 w711 w713 w715 w717 w719 w721 w723 w725 w727 w729 w731 w733 w735 w737 w739 w741 w743 w745 w747 w749 w751 w753 w755 w757 w759 w761 w763 w765 w767 w769 w771 w773 w775 w777 w779 w781 w783 w785 w787 w789 w791 w793 w795 w797 w799 w801]
          tunnel: [w585 w590 w594 w597 w601 w603 w605 w607 w609 w611 w613 w615 w617 w619 w621 w623 w625 w627 w629 w631 w633 w635 w637 w639 w641 w643 w645 w647 w649 w651 w653 w655 w657 w659 w661 w663 w665 w667 w669 w671 w673 w675 w677 w679 w681 w683 w685 w687 w689 w691 w693 w695 w697 w699 w701 w703 w705 w707 w709 w711 w713 w715 w717 w719 w721 w723 w725 w727 w729 w731 w733 w735 w737 w739 w741 w743 w745 w747 w749 w751 w753 w755 w757 w759 w761 w763 w765 w767 w769 w771 w773 w775 w777 w779 w781 w783 w785 w787 w789 w791 w793 w795 w797 w799 w801] -> w535
          tunnel: w511 -> [w587 w589 w593 w599 w600 w602 w604 w606 w608 w610 w612 w614 w616 w618 w620 w622 w624 w626 w628 w630 w632 w634 w636 w638 w640 w642 w644 w646 w648 w650 w652 w654 w656 w658 w660 w662 w664 w666 w668 w670 w672 w674 w676 w678 w680 w682 w684 w686 w688 w690 w692 w694 w696 w698 w700 w702 w704 w706 w708 w710 w712 w714 w716 w718 w720 w722 w724 w726 w728 w730 w732 w734 w736 w738 w740 w742 w744 w746 w748 w750 w752 w754 w756 w758 w760 w762 w764 w766 w768 w770 w772 w774 w776 w778 w780 w782 w784 w786 w788 w790 w792 w794 w796 w798 w800]
          tunnel: [w586 w589 w593 w598 w600 w602 w604 w606 w608 w610 w612 w614 w616 w618 w620 w622 w624 w626 w628 w630 w632 w634 w636 w638 w640 w642 w644 w646 w648 w650 w652 w654 w656 w658 w660 w662 w664 w666 w668 w670 w672 w674 w676 w678 w680 w682 w684 w686 w688 w690 w692 w694 w696 w698 w700 w702 w704 w706 w708 w710 w712 w714 w716 w718 w720 w722 w724 w726 w728 w730 w732 w734 w736 w738 w740 w742 w744 w746 w748 w750 w752 w754 w756 w758 w760 w762 w764 w766 w768 w770 w772 w774 w776 w778 w780 w782 w784 w786 w788 w790 w792 w794 w796 w798 w800] -> w534
          tunnel: w497 -> [w584 w588 w592 w596 _ _ _ _ _ _ _ _ _ _ _ _ _ _ _ _ _ _ _ _ _ _ _ _ _ _ _ _ _ _ _ _ _ _ _ _ _ _ _ _ _ _ _ _ _ _ _ _ _ _ _ _ _ _ _ _ _ _ _ _ _ _ _ _ _ _ _ _ _ _ _ _ _ _ _ _ _ _ _ _ _ _ _ _ _ _ _ _ _ _ _ _ _ _ _ _ _ _ _ _ _]
          frame "DOWN" {
            n1084 = Add(x=w587, y=w584) -> (x+y=w586:sgl)
          }
          frame "LEFT" {
            n1085 = Subtract(x=w591, y=w588) -> (x-y=w590:sgl)
          }
          frame "RIGHT" {
            n1086 = Add(x=w595, y=w592) -> (x+y=w594:sgl)
          }
          frame "UP" {
            n1087 = Subtract(x=w599, y=w596) -> (x-y=w598:sgl)
          }
          frame "ENTER (num pad)" {
          }
          frame "' (quote)" {
          }
          frame "END" {
          }
          frame "EQUALS" {
          }
          frame "ESCAPE" {
          }
          frame "GRAVE (`)" {
          }
          frame "HOME" {
          }
          frame "INSERT" {
          }
          frame "LBRACKET" {
          }
          frame "LCONTROL" {
          }
          frame "L ALT" {
          }
          frame "LSHIFT" {
          }
          frame "LWIN" {
          }
          frame "MINUS" {
          }
          frame "MULTIPLY" {
          }
          frame "NEXT" {
          }
          frame "NUMLOCK" {
          }
          frame "NUMPAD_0" {
          }
          frame "NUMPAD_1" {
          }
          frame "NUMPAD_2" {
          }
          frame "NUMPAD_3" {
          }
          frame "NUMPAD_4" {
          }
          frame "NUMPAD_5" {
          }
          frame "NUMPAD_6" {
          }
          frame "NUMPAD_7" {
          }
          frame "NUMPAD_8" {
          }
          frame "NUMPAD_9" {
          }
          frame "PAUSE" {
          }
          frame "PERIOD" {
          }
          frame "PRIOR (PG UP)" {
          }
          frame "RBRACKET" {
          }
          frame "RCONTROL" {
          }
          frame "RETURN" {
          }
          frame "R ALT" {
          }
          frame "RSHIFT" {
          }
          frame "RWIN" {
          }
          frame "SCROLL" {
          }
          frame "SEMICOLON" {
          }
          frame "SLASH" {
          }
          frame "SPACE" {
          }
          frame "SUBTRACT" {
          }
          frame "TAB" {
          }
          frame "DIVIDE" {
          }
          frame "DELETE" {
          }
          frame "DECIMAL" {
          }
          frame "COMMA" {
          }
          frame "CAPITAL" {
          }
          frame "BACKSLASH" {
          }
          frame "BACK" {
          }
          frame "ADD" {
          }
          frame "F15" {
          }
          frame "F14" {
          }
          frame "F13" {
          }
          frame "F12" {
          }
          frame "F11" {
          }
          frame "F10" {
          }
          frame "F9" {
          }
          frame "F8" {
          }
          frame "F7" {
          }
          frame "F6" {
          }
          frame "F5" {
          }
          frame "F4" {
          }
          frame "F3" {
          }
          frame "F2" {
          }
          frame "F1" {
          }
          frame "Z" {
          }
          frame "Y" {
          }
          frame "X" {
          }
          frame "W" {
          }
          frame "V" {
          }
          frame "U" {
          }
          frame "T" {
          }
          frame "S" {
          }
          frame "R" {
          }
          frame "Q" {
          }
          frame "P" {
          }
          frame "O" {
          }
          frame "N" {
          }
          frame "M" {
          }
          frame "L" {
          }
          frame "K" {
          }
          frame "J" {
          }
          frame "I" {
          }
          frame "H" {
          }
          frame "G" {
          }
          frame "F" {
          }
          frame "E" {
          }
          frame "D" {
          }
          frame "C" {
          }
          frame "B" {
          }
          frame "A" {
          }
          frame "9" {
          }
          frame "8" {
          }
          frame "7" {
          }
          frame "6" {
          }
          frame "5" {
          }
          frame "4" {
          }
          frame "3" {
          }
          frame "2" {
          }
          frame "1" {
          }
          frame "0" {
          }
        }
        n1088 = Bundle(w513, w512, w527, w526, 0.0) -> (w525:cluster{dbl, dbl, dbl, dbl, dbl})  [unwired: 1 in]
        n1089 = Bundle("X"=w535, "Y"=w534) -> (w529:cluster{"X":sgl, "Y":sgl})  [unwired: 1 in]
        n1090 = Divide(x=20, y=w496) -> (x/y=w499:sgl)
        n1091 = property on="Image Out" class="ImageControl"("Image Center Position"=w529) -> ()  [unwired: 2 in, 2 out]
        n1092 = call "IMAQ Convert Rectangle to ROI (Polygon)"("Rectangle"=w525) -> ("ROI Descriptor"=w523:T3)  [unwired: 7 in, 2 out]
        n1093 = Bundle("Application Font", w499, w503, w503, w503, w503, w503, TRUE, w501) -> (w505:T15)  [unwired: 1 in]
        n1094 = property on="Image Out 2" class="ImageControl"("ROI"=w523) -> ()  [unwired: 2 in, 2 out]
        n1095 = Bundle(w501, w505, w501, w501) -> (w504:T16)  [unwired: 1 in]
        n1096 = property on="Image Out" class="ImageControl"() -> ("ROI"=w478:T9)  [unwired: 2 in, 2 out]
        n1097 = Unbundle By Name(w478) -> ("Contours"=w552:T12)
        n1098 = local read "Image Out"() -> (w507:T2)
        n1099 = call "IMAQ Clear Overlay"("Image"=w507) -> ("Image Out"=w506:T2)  [unwired: 9 in, 1 out]
        n1100 = Initialize Array(0) -> (w550:i32[])  [unwired: 1 in]
        n1101 = local read "Magnification"() -> (w541:u16)
        n1102 = Array Size(array=w552) -> (size(s)=w551:i32)
        n1103 = Build Array(0.505025, 0.252522, 0.127742, 0.050345, 0.031129) -> (w542:dbl[])
        n1104 = Array Subset(array=w542, index=w541, length=1) -> (w539:dbl[])
        n1105 = property on="Image Out" class="ImageControl"() -> ("ZoomInteger"=w531:cluster{"X":i32, "Y":i32})  [unwired: 2 in, 2 out]
        n1106 = To Double Precision Float(number=w539) -> (double precision float=w538:dbl[])
        n1107 = for {
          N: w551 -> [_]
          shift-right: [w824] -> _
          shift-left: w552 -> [w824]
          shift-right: [w822] -> w537
          shift-left: w550 -> [w821]
          tunnel: w538 -> [w820]
          shift-right: [w817] -> _
          shift-left: w506 -> [w819]
          tunnel: w504 -> [w812]
          i -> [w816]
          n1108 = Index Array(array=w824, index=w816) -> (element=w833:T17)
          n1109 = Unbundle(w833) -> ("Points"=w832:i32[])  [unwired: 2 out]
          n1110 = Array To Cluster(array=w832) -> (cluster=w831:T18)
          n1111 = Unbundle(w831) -> ("Points[0]"=w811:i32, "Points[1]"=w808:i32, "Points[2]"=w823:i32, "Points[3]"=w829:i32)  [unwired: 5 out]
          n1112 = Add(x=w811, y=10) -> (x+y=w809:i32)
          n1113 = Subtract(x=w808, y=w829) -> (x-y=w828:i32)
          n1114 = Subtract(x=w811, y=w823) -> (x-y=w830:i32)
          n1115 = Square(x=w828) -> (x^2=w826:i32)
          n1116 = Square(x=w830) -> (x^2=w827:i32)
          n1117 = Add(x=w827, y=w826) -> (x+y=w825:i32)
          n1118 = Square Root(x=w825) -> (sqrt(x)=w802:dbl)
          n1119 = Multiply(x=w802, y=0.5) -> (x*y=w805:dbl)
          n1120 = Add(x=w805, y=w808) -> (x+y=w807:dbl)
          n1121 = Bundle(w809, w807) -> (w818:cluster{i32, dbl})  [unwired: 1 in]
          n1122 = Multiply(x=w802, y=w820) -> (x*y=w815:dbl[])
          n1123 = Index Array(array=w815) -> (element=w814:dbl)  [unwired: 1 in]
          n1124 = Number To Fractional String(number=w814) -> (F-format string=w813:string)  [unwired: 3 in]
          n1125 = call "IMAQ Overlay Text"("BG Color (Transparent)"=u32 0, "Text Color (black)"=u32 16448250, "Font, Size & Style"=w812, "String"=w813, "Origin"=w818, "Image"=w819) -> ("Image Out"=w817:T2)  [unwired: 4 in, 1 out]
          n1126 = Build Array (concatenate)(w821, w815) -> (w822:dbl[])
          n1127 = local write "Numeric 3"(w802) -> ()
        }
        n1128 = local write "ROI Descriptor"(w478) -> ()
        n1129 = Unbundle(w531) -> ("X"=w530:i32)  [unwired: 1 out]
        n1130 = Add Array Elements(numeric array=w537) -> (sum=w548:dbl)
        n1131 = local write "Distances"(w537) -> ()
        n1132 = local write "Total Width"(w548) -> ()
        n1133 = local write "Zoom"(w530) -> ()
        n1134 = local read "Rec: Width"() -> (w479:dbl)
        n1135 = local read "Manual"() -> (w477:bool)
        n1136 = Not(x=w477) -> (.not. x?=w475:bool)
        n1137 = local read "Total Width"() -> (w481:dbl)
        n1138 = Equal To 0?(x=w481) -> (x = 0?=w476:bool)
        n1139 = And(x=w476, y=w475) -> (x .and. y?=w474:bool)
        n1140 = case shown="True" w474 {
          tunnel: w479 -> [_ w562]
          frame False {
          }
          frame True {
            n1141 = local write "New: Width"(w562) -> ()
          }
        }
        n1142 = Or(x=w476, y=w477) -> (x .or. y?=w480:bool)
        n1143 = case shown="False" w480 {
          tunnel: w481 -> [w563 _]
          frame False {
            n1144 = local write "New: Width"(w563) -> ()
          }
          frame True {
          }
        }
      }
    }
  }
  n1145 = Build Array("DeviceID", "Fabricator", "Deposition", "Date", "Sample", "Row", "Column", "L (um)", "W (um)", "Material", "Treatment", "TC (mM)", "Solvent", "C (%)", "ST (C)", "Drops", "Wait (s)", "RT (F)", "RH (%)", "Ramp (s)", "RPM", "Accel (RPM/s)", "Time (s)", "Mobility", "On/Off", "Vt", "S.T.S") -> (→"Transformer \nHeaders":string[])
